vi "lightsheetMain_changeLasers.vi"() -> ()   [LabVIEW 2015]
panel:
  in  "initLaserPower":dbl=2.0
  out "initLasers":T1(array[cluster])=[{"Component ID"="405nm", "COM Port"="COM14", "Type "=enum."omicronLuxX", "init"=1, "Max power (mW)"=60.0}, {"Component ID"="488nm", "COM Port"="COM4", "Type "=enum."omicronLuxX", "init"=1, "Max power (mW)"=60.0}, {"Component ID"="561nm", "COM Port"="COM27", "Type "=enum."coherentObis", "init"=1, "Max power (mW)"=50.0}, {"Component ID"="642nm", "COM Port"="COM12", "Type "=enum."omicronLuxX", "init"=1, "Max power (mW)"=140.0}]
  out "acquisitionTime":u32
  out "opticalSectionThickness (um)":dbl=5.0
  out "acqLaserCOM":refnum<visa-resource-name>[](array[refnum])
  out "acqLaserOff":string[](array[string])
  out "acqLaserOn":string[](array[string])
  out "acqFW":u8[](array[numeric])
  out "Lat x inc (mm)":dbl=0.37273599999999996
  out "Lat y inc (mm)":dbl=0.37273599999999996
  out "no y steps":i32=1
  out "no colours":i32=1
  out "no z imgs (acq)":i32=1
  out "no x steps":i32=1
  out "stop live view":bool
  out "LH yLim (mm)":dbl
  out "RH yLim (mm)":dbl
  in  "Set RH yLim":bool
  in  "Set LH yLim":bool
  out "TH zLim (mm)":dbl
  in  "Set TH zLim":bool
  in  "acqLSFM_3":enum32{"Acquisition (hardware)"}(tab)
  out "Generating tiff stacks":bool
  out "Acquisition in progress":bool
  in  "convertDcimgToTifStacks":bool=TRUE
  in  "setupAcq":bool
  in  "testAcq":bool
  out "x1":dbl
  out "y1":dbl
  out "z1":dbl
  out "x2":dbl
  out "y2":dbl
  out "z2":dbl
  in  "no z steps":i32=1
  in  "% FOV overlap":i32=10
  in  "z inc (um)":dbl=1.0
  in  "642":bool=TRUE
  in  "561":bool=TRUE
  in  "405":bool=TRUE
  in  "488":bool=TRUE
  in  "beginAcq":bool
  in  "stopAcq":bool
  in  "end all comms and exit":bool
  in  "acquisitionMode":enum32{"stop/start  ", "cont."}(radio)
  out "z inc (mm)":dbl=0.01
  in  "Save acq vals":bool
  in  "Read acq vals":bool
  out "Filter wheel":cluster{"FW Handle":u32, "init?":i16}={"FW Handle"=428794912, "init?"=1}
  out "sCMOS":cluster{"init":i16, "sCMOS handle":u32}
  out "Z stage":T2={"System no."=2, "zIdx"=1, "zLim (mm)"=0.0, "0, 1"=0}
  out "XY stage":T3={"System no."=1, "xIdx"=1, "yIdx"=2, "xLim (mm)"=0.0, "yLim (mm)"=0.0, "0, 1"=0}
  in  "LSFM_3":T4(tab)=enum."lasers/filters"
  out "acqDelay (ms)":u32=10
  out "fine axial vel (mm/s)":dbl=10.0
  in  "set axial vel":bool
  in  "filename":string="testImg"
  in  "Index":i32
  in  "Down":bool
  in  "Up":bool
  in  "Left":bool
  in  "Right":bool
  in  "Backward":bool
  in  "Forward":bool
  in  "Axial stepsize (mm/um)":dbl=1.0
  in  "Lateral stepsize (mm/um)":dbl=1.0
  in  "Toggle coarse/fine":enum32{"Coarse (mm) ", "Fine (um) "}(radio)
  out "x (mm)":dbl
  out "y (mm)":dbl
  out "z (mm)":dbl
  in  "Snap img":bool
  in  "set init xy pos":bool
  in  "set fin xy pos":bool
  in  "set init z":bool
  in  "set fin z":bool
  in  "mov init xy":bool
  in  "mov init z":bool
  in  "mov fin xy":bool
  in  "mov fin z":bool
  in  "coarse axial vel (mm/s)":dbl=6.0
  in  "642 nm power (mW)":dbl(slide)=54.0 min=0.0 max=60.0 step=1.0 scale=0.0..140.0
  in  "561 nm power (mW)":dbl(slide)=8.0 min=0.0 max=60.0 step=1.0 scale=0.0..60.0
  in  "488 nm power (mW)":dbl(slide)=5.0 min=0.0 max=60.0 step=1.0 scale=0.0..60.0
  in  "405 nm power (mW)":dbl(slide)=5.0 min=0.0 max=60.0 step=1.0 scale=0.0..60.0
  in  "FW pos":u16(ring)=4 items=["460/36 [DAPI]"=1, "525/50 [FITC]"=2, "605/70 [Cy3]"=3, "665/LP [Cy5]"=4, "Empty-1"=5, "Empty-2"=6]
  in  "next":bool
  in  "prev":bool
  in  "642 nm ON":bool
  in  "642 nm OFF":bool
  in  "561 nm ON":bool
  in  "561 nm OFF":bool
  in  "488 nm ON":bool
  in  "488 nm OFF":bool
  in  "405 nm ON":bool
  in  "405 nm OFF":bool
  in  "405 filter":u8(ring)=1 items=["460/36 [DAPI]"=1, "525/50 [FITC]"=2, "605/70 [Cy3]"=3, "665/LP [Cy5]"=4, "Empty-1"=5, "Empty-2"=6]
  in  "488 filter":u8(ring)=2 items=["460/36 [DAPI]"=1, "525/50 [FITC]"=2, "605/70 [Cy3]"=3, "665/LP [Cy5]"=4, "Empty-1"=5, "Empty-2"=6]
  in  "561 filter":u8(ring)=3 items=["460/36 [DAPI]"=1, "525/50 [FITC]"=2, "605/70 [Cy3]"=3, "665/LP [Cy5]"=4, "Empty-1"=5, "Empty-2"=6]
  in  "642 filter":u8(ring)=4 items=["460/36 [DAPI]"=1, "525/50 [FITC]"=2, "605/70 [Cy3]"=3, "665/LP [Cy5]"=4, "Empty-1"=5, "Empty-2"=6]
  out "Acquiring?":bool
  in  "live stream":bool
  in  "Set exp. time":bool
  in  "Exposure time (s)":dbl=1.0
  in  "stop live stream":bool
  in  "View stream":bool=TRUE
  out "Img. pixel size":dbl=0.26
  out "No. of pix":u16=2048
  in  "pixel binning":u16(ring) items=["1x1"=1, "2x2"=2, "4x4"=4]
  in  "No. pix":u16=2048
  in  "scmos pixel size (um)":dbl=6.5 format="%#_13g"
  out "FOV (mm)":dbl=0.53248
  in  "sensorSize":dbl=13.312 format="%#_13g"
  in  "Mag":dbl=25.0 format="%#_13g"
  in  "z":bool
  in  "xy":bool
  in  "488nm":bool=TRUE
  in  "405nm":bool=TRUE
  in  "561nm":bool=TRUE
  in  "642nm":bool=TRUE
  in  "sCMOS":bool
  in  "FW":bool=TRUE
  out "Appended path":path=path "C:/Users/LSFM_2/Desktop/dataAcq_2705/bothIllAxis/4umBead0.tif"
  in  "Base path":path=path "C:/Users/sims01/Desktop/dataAcq"
  in  "dcimgToStack":bool
  in  "stageAccDelay (ms)":u32
  # "Stage limits"
  # "Positions"
  # "Step sizes"
  # "Currrent positions"
  # "Motion control"
  # "Move stages"
  # "lasers"
  # "filters"
  # "File setup"
  # "Hardware initialization"
  # "Microscope properties"
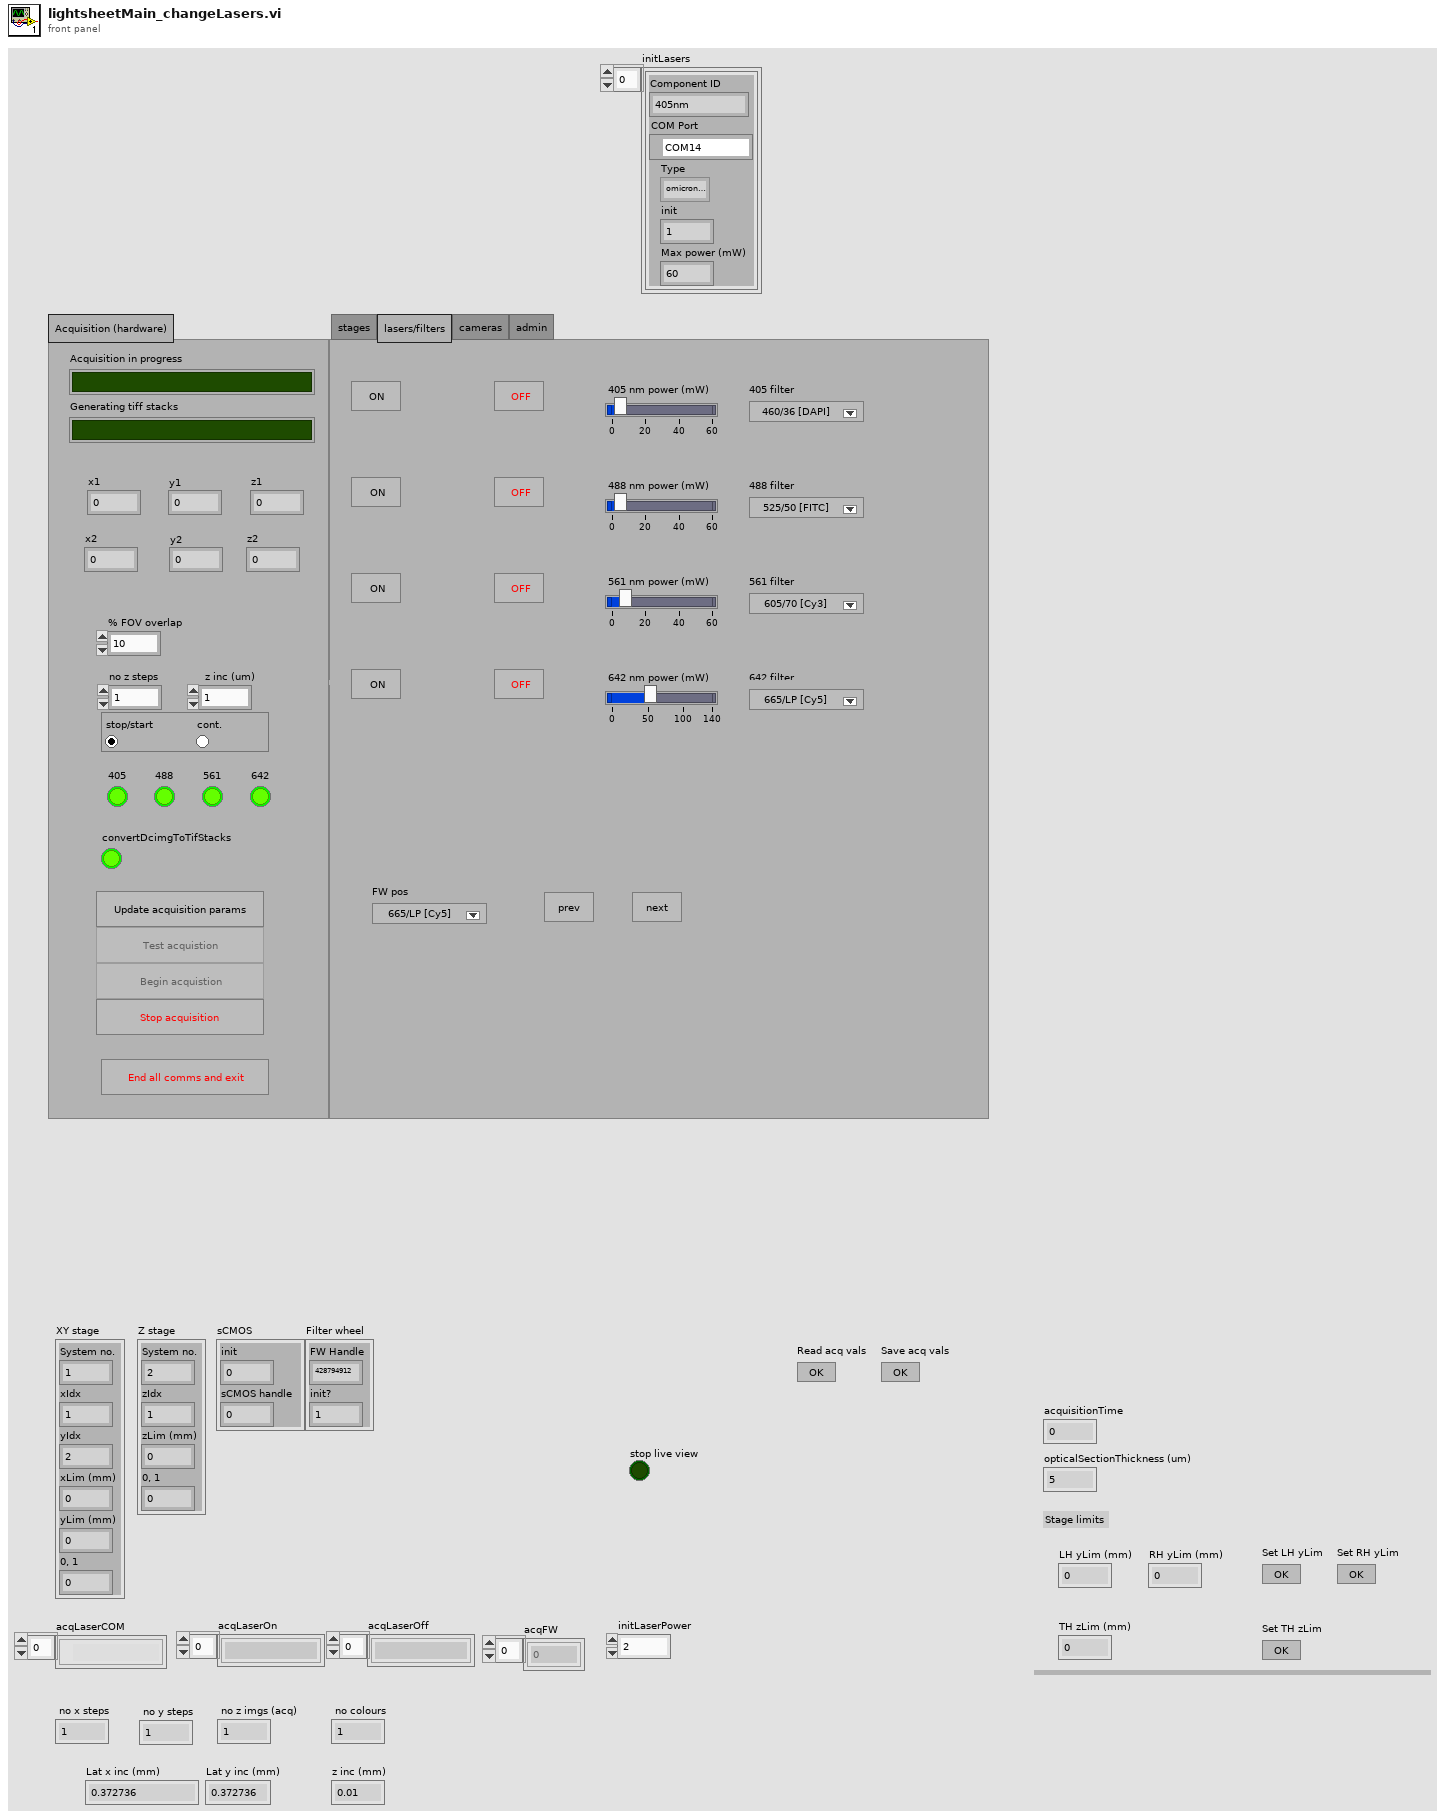
[diagram p1: front panel]
types:
  T1 = cluster{"Component ID":string, "COM Port":refnum<visa-resource-name>, "Type ":enum16{"omicronLuxX", "coherentObis"}, "init":i16, "Max power (mW)":dbl}[]
  T2 = cluster{"System no.":i32, "zIdx":i32, "zLim (mm)":dbl, "0, 1":i16}
  T3 = cluster{"System no.":i32, "xIdx":i32, "yIdx":i32, "xLim (mm)":dbl, "yLim (mm)":dbl, "0, 1":i16}
  T4 = enum32{"stages", "lasers/filters", "cameras", "admin"}
  T5 = enum8{"Enabled", "Disabled", "Disabled and Grayed Out"}
  T6 = cluster{"Component ID":string, "COM Port":refnum<visa-resource-name>, "Type ":enum16{"omicronLuxX", "coherentObis"}, "init":i16, "Max power (mW)":dbl}
  T7 = enum32{"Invalid", "Standard", "Closed", "Hidden", "Minimized", "Maximized"}
  T8 = cluster{"height":u32, "width":u32, "datatype":u32}
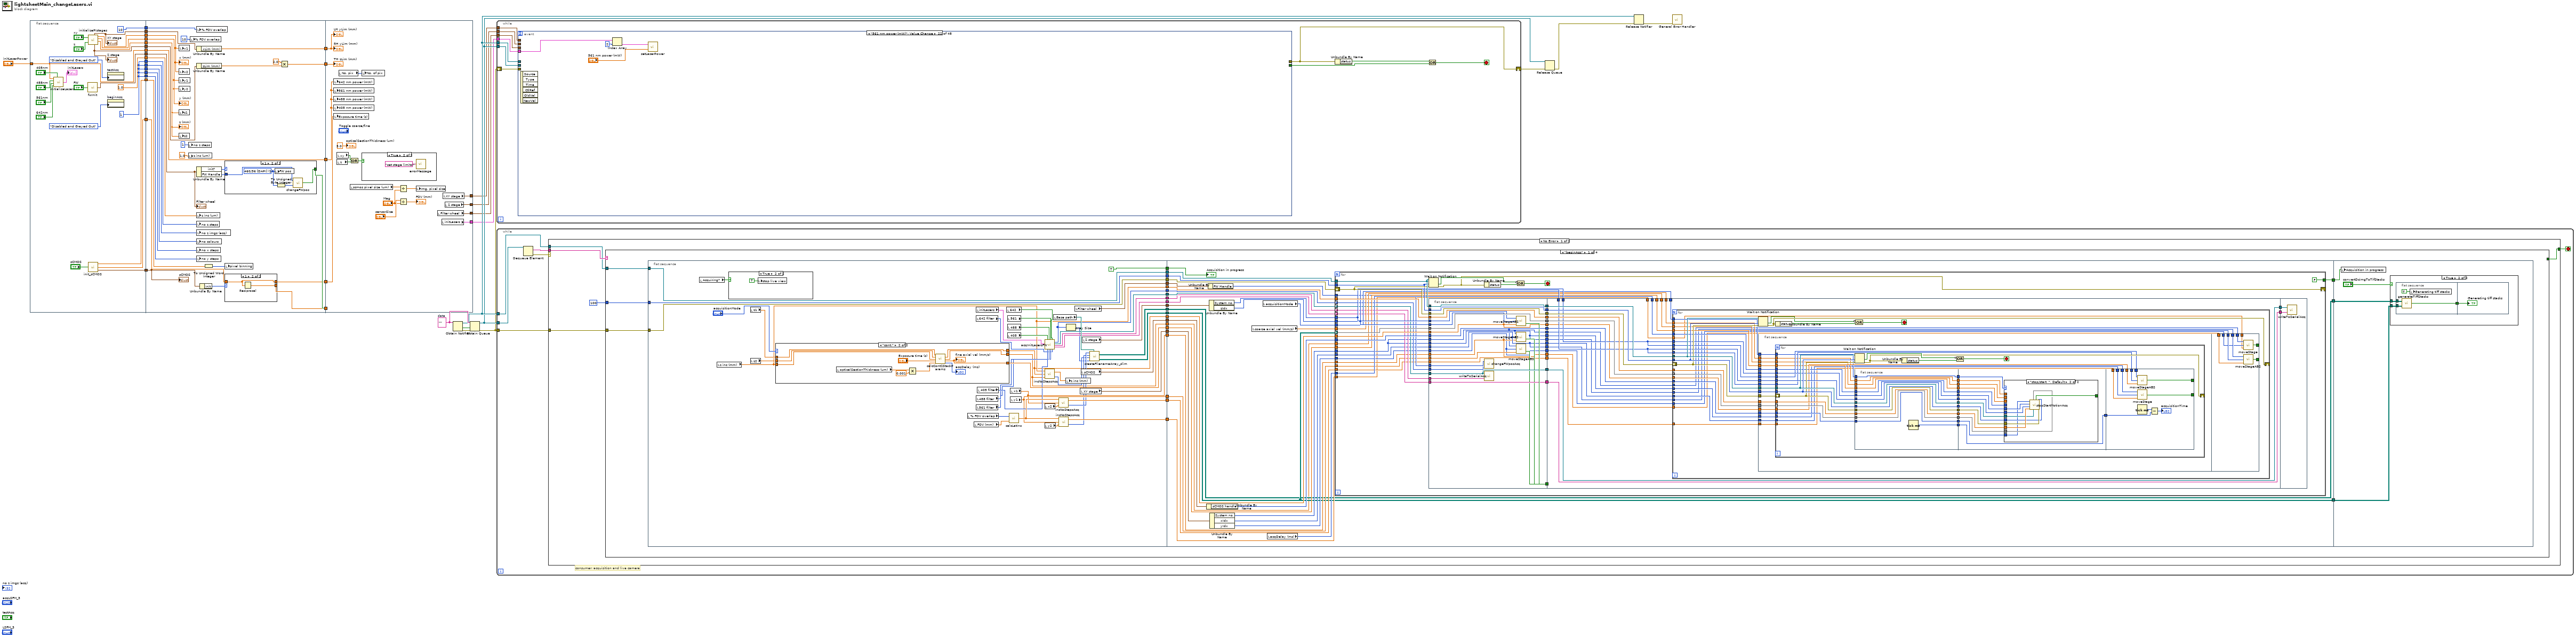
[diagram p0: block diagram]
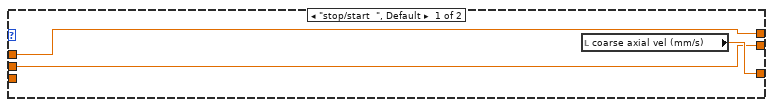
[diagram p3: hidden frame]
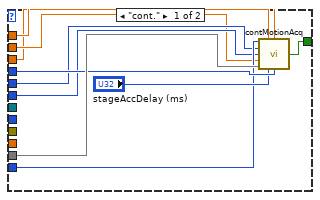
[diagram p4: hidden frame]
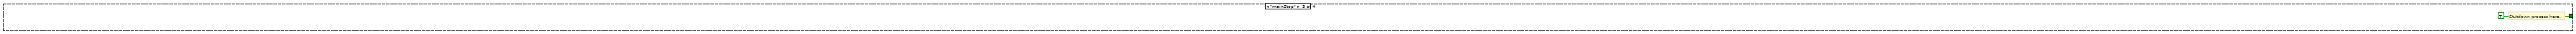
[diagram p7: hidden frame]
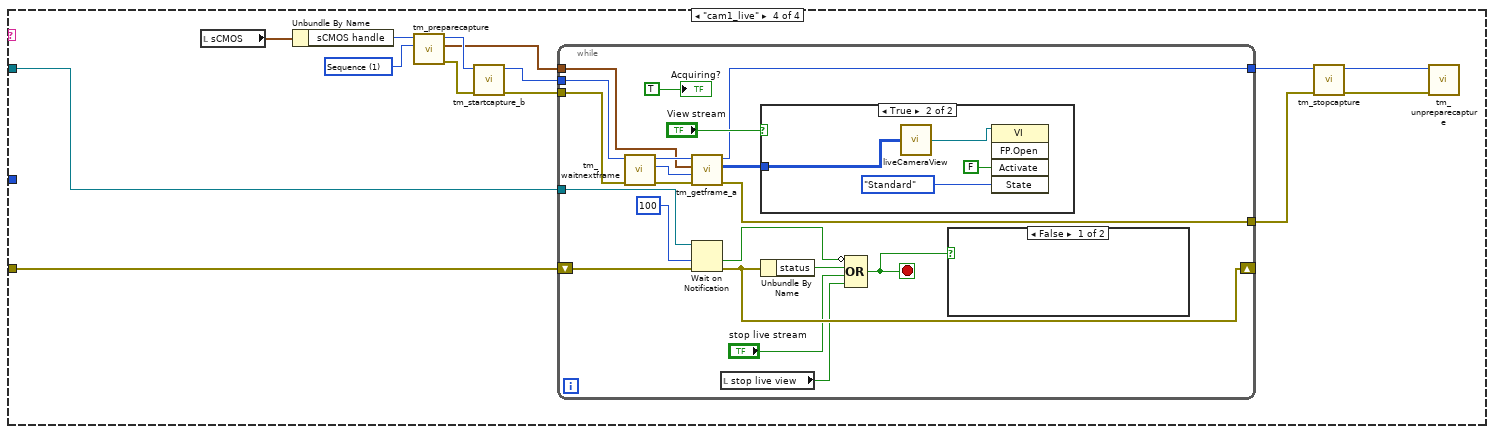
[diagram p8: hidden frame]
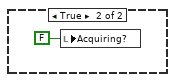
[diagram p9: hidden frame]
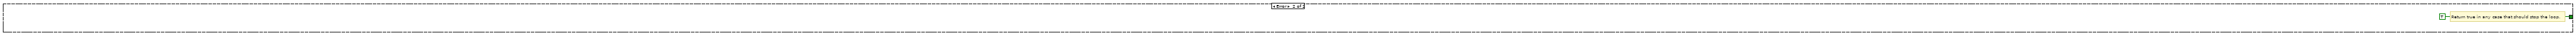
[diagram p11: hidden frame]
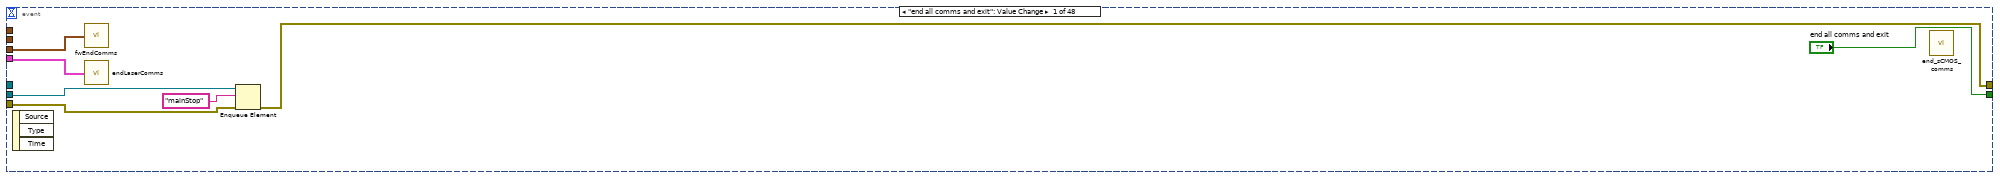
[diagram p12: hidden frame]
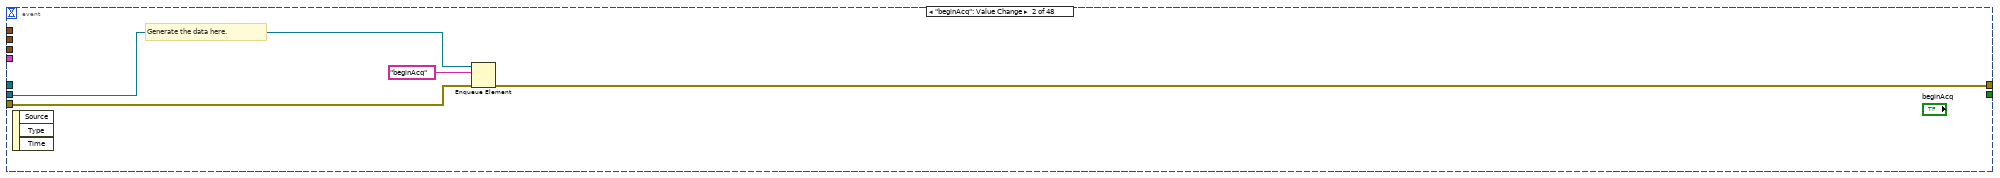
[diagram p13: hidden frame]
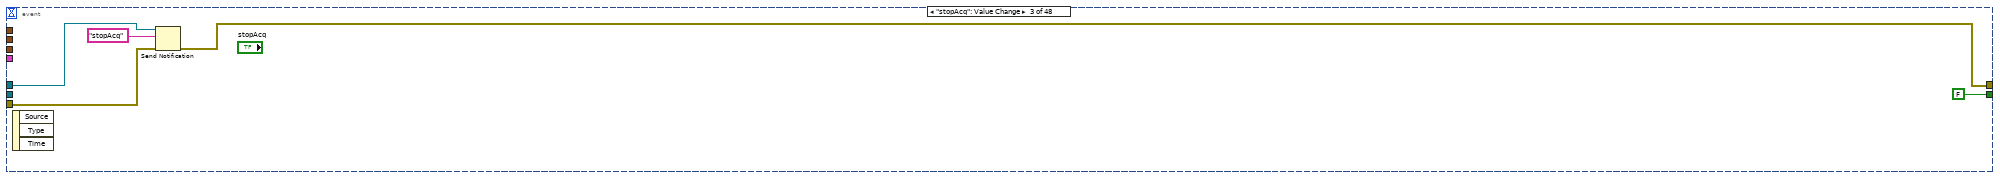
[diagram p14: hidden frame]
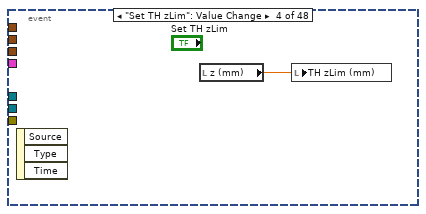
[diagram p15: hidden frame]
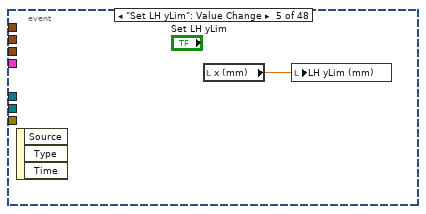
[diagram p16: hidden frame]
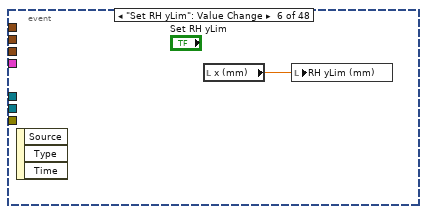
[diagram p17: hidden frame]
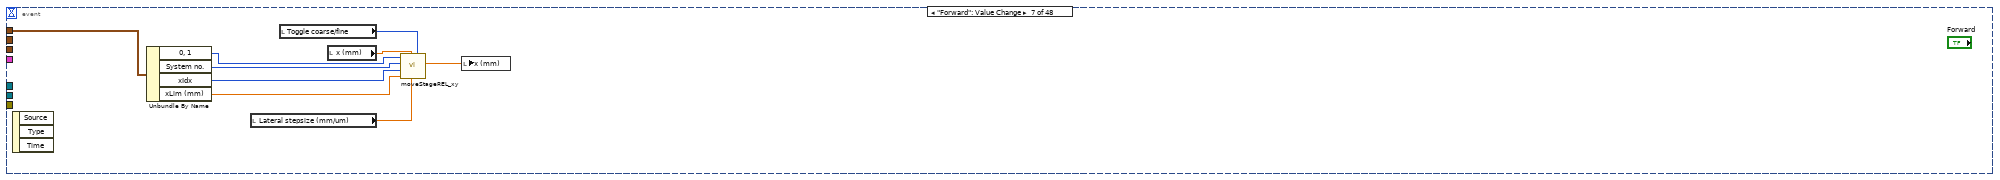
[diagram p18: hidden frame]
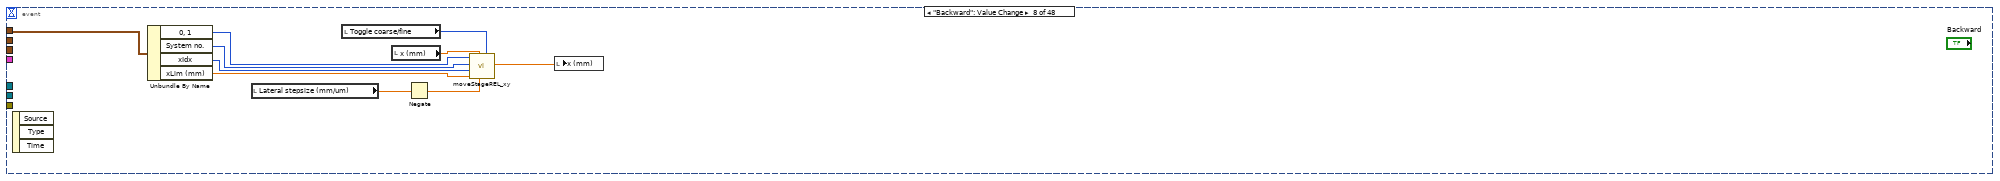
[diagram p19: hidden frame]
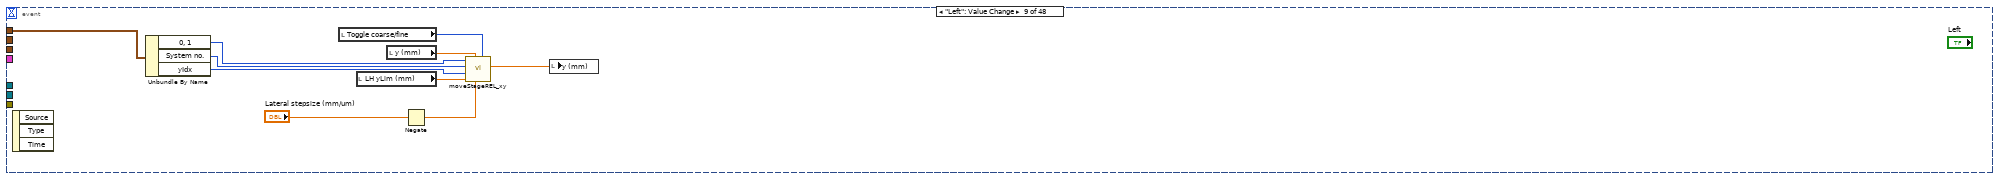
[diagram p20: hidden frame]
diagram:
  w26 = ""  # data
  n1 = flat-sequence {
    tunnel: [w59] -> w37
    tunnel: [w58] -> w36
    tunnel: [w57] -> w35
    tunnel: [w50] -> w34
    tunnel: [w49] -> w33
    tunnel: [w56] -> w32
    tunnel: [w55] -> w16
    tunnel: [w54] -> w15
    tunnel: [w48] -> w11
    tunnel: [w46] -> w10
    tunnel: [w46] -> w9
    tunnel: [w46] -> w8
    tunnel: [w46] -> w7
    tunnel: [10 ("% FOV overlap")] -> w6
    tunnel: [w46] -> w5
    tunnel: [1.0 ("z inc (um)")] -> w4
    tunnel: "initLaserPower" -> [w38]
    tunnel: [w38] -> w1
    tunnel: w37 -> [w75]
    tunnel: w36 -> [w76]
    tunnel: w35 -> [w77]
    tunnel: w34 -> [w90]
    tunnel: w33 -> [w92]
    tunnel: w32 -> [w89]
    tunnel: [w86] -> w31
    tunnel: [w85] -> w30
    tunnel: [w84] -> w29
    tunnel: w16 -> [w83]
    tunnel: w15 -> [w82]
    tunnel: [w81] -> w14
    tunnel: [w80] -> w13
    tunnel: w11 -> [w71]
    tunnel: w10 -> [w70]
    tunnel: w9 -> [w69]
    tunnel: w8 -> [w68]
    tunnel: w7 -> [w67]
    tunnel: w6 -> [w66]
    tunnel: w5 -> [w65]
    tunnel: w4 -> [w64]
    tunnel: [w62] -> w3
    tunnel: w1 -> [w62]
    tunnel: w31 -> [_]
    tunnel: w30 -> [w113]
    tunnel: w29 -> [_]
    tunnel: [w112] -> w18
    tunnel: [w111] -> w17
    tunnel: [w110] -> w19
    tunnel: w14 -> [w109]
    tunnel: w13 -> [w108]
    tunnel: [w102] -> w12
    tunnel: w3 -> [w101]
    frame #0 {
      w46 = 1 ("no y steps")
      n2 = call "initialiseLasers.vi"("initLaserPower"=w38, "488 nm"="488nm", "561 nm"="561nm", "642 nm"="642nm", "405 nm"="405nm") -> ("outputLasers"=→"initLasers":T1)
      n3 = call "fwInit.vi"("FW init?"="FW") -> ("Filter wheel init"=w56:cluster{"FW Handle":u32, "init?":i16})
      n4 = call "initializePIstages.vi"("xy stage"="xy", "z stage"="z") -> ("XY stage"=w54:T3, "Z stage"=w55:T2, "current xPos (mm)"=w59:dbl, "current yPos (mm)"=w58:dbl, "current zPos (mm)"=w57:dbl)  [unwired: 1 in]
      "XY stage" <- w54
      "Z stage" <- w55
      n5 = call "init_sCMOS.vi"("sCMOS_1"="sCMOS") -> ("Binning"=w48:dbl, "Exposure"=w50:dbl, "sCMOS init"=w49:cluster{"init":i16, "sCMOS handle":u32})
      n6 = property on="testAcq" class="Bool"("DisabledEnum"=T5."Disabled and Grayed Out" ("Disabled")) -> ()  [unwired: 2 in, 2 out]
      n7 = property on="beginAcq" class="Bool"("DisabledEnum"=T5."Disabled and Grayed Out" ("Disabled")) -> ()  [unwired: 2 in, 2 out]
    }
    frame #1 {
      n8 = local write "x1"(w75) -> ()
      n9 = local write "x2"(w75) -> ()
      n10 = local write "y1"(w76) -> ()
      n11 = local write "y2"(w76) -> ()
      n12 = local write "z1"(w77) -> ()
      n13 = local write "z2"(w77) -> ()
      n14 = local write "no z steps"(1 ("no z steps")) -> ()
      n15 = local write "z inc (um)"(1.0 ("z inc (um)")) -> ()
      n16 = local write "% FOV overlap"(10 ("% FOV overlap")) -> ()
      n17 = local write "% FOV overlap"(w66) -> ()
      n18 = Unbundle By Name(w82) -> ("xLim (mm)"=w81:dbl)
      n19 = Unbundle By Name(w83) -> ("zLim (mm)"=w79:dbl)
      n20 = Unbundle By Name(w89) -> ("init?"=w88:i16, "FW Handle"=w87:u32)
      n21 = local write "z inc (um)"(w64) -> ()
      n22 = local write "no z steps"(w65) -> ()
      n23 = local write "no z imgs (acq)"(w68) -> ()
      n24 = local write "no colours"(w69) -> ()
      n25 = local write "no x steps"(w67) -> ()
      n26 = local write "no y steps"(w70) -> ()
      n27 = Unbundle By Name(w92) -> ("init"=w91:i16)
      n28 = To Unsigned Word Integer(number=w71) -> (unsigned 16bit integer=w72:u16)
      n29 = case shown="1" w88 {
        tunnel: w87 -> [_ w97]
        tunnel: [FALSE ("fwPosChanged") w96] -> w86
        frame 0, Default {
        }
        frame 1 {
          w94 = u16 1 items=["460/36 [DAPI]"=1, "525/50 [FITC]"=2, "605/70 [Cy3]"=3, "665/LP [Cy5]"=4, "Empty-1"=5, "Empty-2"=6] ("Filter wheel position")
          n30 = local write "FW pos"(w94) -> ()
          n31 = To Unsigned Byte Integer(number=w94) -> (unsigned 8bit integer=w95:u8)
          n32 = call "changeFWpos.vi"("FW pos"=w95, "FWhandle"=w97) -> ("fwPosChanged"=w96:bool)
        }
      }
      n33 = local write "pixel binning"(w72) -> ()
      n34 = case shown="1" w91 {
        tunnel: w90 -> [_ w100]
        tunnel: [w98 w100] -> w85
        tunnel: [w98 w99] -> w84
        frame 0, Default {
          w98 = 1.0
        }
        frame 1 {
          n35 = Reciprocal(x=w100) -> (1/x=w99:dbl)
        }
      }
      n36 = Multiply(x=2.0, y=w79) -> (x*y=w80:dbl)
      "z (mm)" <- w77
      "y (mm)" <- w76
      "x (mm)" <- w75
      "sCMOS" <- w92
      "Filter wheel" <- w89
    }
    frame #2 {
      n37 = local write "642 nm power (mW)"(w101) -> ()
      n38 = local write "561 nm power (mW)"(w101) -> ()
      n39 = local write "488 nm power (mW)"(w101) -> ()
      n40 = local write "405 nm power (mW)"(w101) -> ()
      n41 = local write "Exposure time (s)"(w113) -> ()
      n42 = local read "xy"() -> (w115:bool)
      n43 = local read "z"() -> (w114:bool)
      n44 = local read "No. pix"() -> (w104:u16)
      n45 = Or(x=w115, y=w114) -> (x .or. y?=w116:bool)
      n46 = local read "scmos pixel size (um)"() -> (w106:dbl)
      n47 = local write "No. of pix"(w104) -> ()
      n48 = case shown="True" w116 {
        frame False {
        }
        frame True {
          n49 = call "errorMessage.vi"("messageText"="set stage limits!") -> ()  [unwired: 3 out]
        }
      }
      n50 = Divide(x=w106, y="Mag") -> (x/y=w105:dbl)
      n51 = Divide(x="sensorSize", y="Mag") -> (x/y=→"FOV (mm)":dbl)
      n52 = local write "Img. pixel size"(w105) -> ()
      n53 = local read "Filter wheel"() -> (w112:cluster{"FW Handle":u32, "init?":i16})
      n54 = local read "initLasers"() -> (w102:T1)
      n55 = local read "XY stage"() -> (w111:T3)
      n56 = local read "Z stage"() -> (w110:T2)
      "TH zLim (mm)" <- w108
      "RH yLim (mm)" <- w109
      "LH yLim (mm)" <- w109
      "opticalSectionThickness (um)" <- 5.0 ("opticalSectionThickness (um)")
    }
  }
  n57 = Obtain Notifier(notification data type=w26) -> (notifier out=w22:refnum<notifier>, created new?=w28:bool, error out=w27:errorcluster)  [unwired: 3 in]
  n58 = Obtain Queue(element data type=w26, create if not found? (T)=w28, error in (no error)=w27) -> (queue out=w21:refnum<queue>, error out=w20:errorcluster)  [unwired: 2 in, 1 out]
  n59 = while {
    shift-right: [w126] -> w25
    shift-left: w20 -> [w129]
    tunnel: w21 -> [w130]
    tunnel: w22 -> [w124]
    tunnel: w19 -> [w123]
    tunnel: w18 -> [w122]
    tunnel: w17 -> [w121]
    tunnel: w12 -> [w120]
    stop <- w127 stop-if-true
    n60 = event shown="[21] \"561 nm power (mW)\": Value Change" {
      selector: _ -> [_ _ _ _ _ _ _ _ _ _ _ _ _ _ _ _ _ _ _ _ _ _ _ _ _ _ _ _ _ _ _ _ _ _ _ _ _ _ _ _ _ _ _ _ _ _ _ _]
      dyn-events: _ -> [_ _ _ _ _ _ _ _ _ _ _ _ _ _ _ _ _ _ _ _ _ _ _ _ _ _ _ _ _ _ _ _ _ _ _ _ _ _ _ _ _ _ _ _ _ _ _ _]
      timeout: _ -> [_ _ _ _ _ _ _ _ _ _ _ _ _ _ _ _ _ _ _ _ _ _ _ _ _ _ _ _ _ _ _ _ _ _ _ _ _ _ _ _ _ _ _ _ _ _ _ _]
      tunnel: w130 -> [w134 w141 _ _ _ _ _ _ _ _ _ _ _ _ _ _ _ _ _ _ _ _ _ _ _ _ _ _ _ w306 _ _ _ _ _ _ _ _ _ _ _ _ _ _ _ _ _ _]
      tunnel: w129 -> [w136 w140 w146 _ _ _ _ _ _ _ _ _ _ _ _ _ _ _ _ _ _ _ _ _ _ _ _ _ _ w308 _ _ _ _ _ _ _ _ _ _ _ _ _ _ _ _ _ _]
      tunnel: [w135 w139 w145 _ _ _ _ _ _ _ _ _ _ _ _ _ _ _ _ _ _ _ _ _ _ _ _ _ _ w307 _ _ _ _ _ _ _ _ _ _ _ _ _ _ _ _ _ _] -> w126
      tunnel: ["end all comms and exit" _ FALSE ("stop") _ _ _ _ _ _ _ _ _ _ _ _ _ _ _ _ _ _ _ _ _ _ _ _ _ _ _ _ _ _ _ _ _ _ _ _ _ _ _ _ _ _ _ _ _] -> w128
      tunnel: w124 -> [_ _ w144 _ _ _ _ _ _ _ _ _ _ _ _ _ _ _ _ _ _ _ _ _ _ _ _ _ _ _ _ _ _ _ _ _ _ _ _ _ _ _ _ _ _ _ _ _]
      tunnel: w123 -> [_ _ _ _ _ _ _ _ _ _ w196 w206 w208 _ _ _ _ _ _ _ _ _ _ _ _ _ _ _ _ _ _ _ _ _ _ _ _ _ _ w376 w380 _ _ _ _ _ w417 _]
      tunnel: w122 -> [w131 _ _ _ _ _ _ _ _ _ _ _ _ w211 _ _ w224 _ _ w240 _ _ w255 _ _ w271 w277 w288 _ _ _ _ _ _ _ _ _ _ _ _ _ _ _ _ _ _ w418 _]
      tunnel: w121 -> [_ _ _ _ _ _ w158 w168 w178 w187 _ _ _ _ _ _ _ _ _ _ _ _ _ _ _ _ _ _ _ _ _ _ _ _ _ w355 w356 _ _ _ _ _ _ _ _ _ w416 _]
      tunnel: w120 -> [w132 _ _ _ _ _ _ _ _ _ _ _ _ w213 w217 w222 w228 w232 w237 w243 w247 w252 w258 w262 w267 _ _ _ _ _ _ _ _ _ _ _ _ _ _ _ _ _ _ _ _ _ w414 _]
      event "end all comms and exit": Value Change {
        n61 = event-data() -> ()  [unwired: 1 in, 3 out]
        n62 = call "fwEndComms.vi"("fw cluster"=w131) -> ()
        n63 = call "endLaserComms.vi"("outputLasers"=w132) -> ()
        n64 = Enqueue Element(queue=w134, element="mainStop", error in (no error)=w136) -> (error out=w135:errorcluster)  [unwired: 1 in, 2 out]
        n65 = call "end_sCMOS_comms.vi"() -> ()  [unwired: 1 in]
      }
      event "beginAcq": Value Change {
        # "Generate the data here."
        n66 = event-data() -> ()  [unwired: 1 in, 3 out]
        n67 = Enqueue Element(queue=w141, element="beginAcq", error in (no error)=w140) -> (error out=w139:errorcluster)  [unwired: 1 in, 2 out]
      }
      event "stopAcq": Value Change {
        n68 = event-data() -> ()  [unwired: 1 in, 3 out]
        n69 = Send Notification(notification="stopAcq", notifier=w144, error in (no error)=w146) -> (error out=w145:errorcluster)  [unwired: 1 out]
      }
      event "Set TH zLim": Value Change {
        n70 = event-data() -> ()  [unwired: 1 in, 3 out]
        n71 = local read "z (mm)"() -> (w147:dbl)
        n72 = local write "TH zLim (mm)"(w147) -> ()
      }
      event "Set LH yLim": Value Change {
        n73 = event-data() -> ()  [unwired: 1 in, 3 out]
        n74 = local read "x (mm)"() -> (w148:dbl)
        n75 = local write "LH yLim (mm)"(w148) -> ()
      }
      event "Set RH yLim": Value Change {
        n76 = event-data() -> ()  [unwired: 1 in, 3 out]
        n77 = local read "x (mm)"() -> (w149:dbl)
        n78 = local write "RH yLim (mm)"(w149) -> ()
      }
      event "Forward": Value Change {
        n79 = event-data() -> ()  [unwired: 1 in, 3 out]
        n80 = Unbundle By Name(w158) -> ("0, 1"=w157:i16, "System no."=w156:i32, "xIdx"=w155:i32, "xLim (mm)"=w154:dbl)
        n81 = local read "Lateral stepsize (mm/um)"() -> (w153:dbl)
        n82 = local read "Toggle coarse/fine"() -> (w151:enum32{"Coarse (mm) ", "Fine (um) "})
        n83 = local read "x (mm)"() -> (w152:dbl)
        n84 = call "moveStageREL_xy.vi"("Radio Buttons"=w151, "increment"=w153, "initPos (mm)"=w152, "stage lim (mm)"=w154, "axisIdx"=w155, "System no."=w156, "stageInit"=w157) -> ("finPos"=w150:dbl)  [unwired: 3 in]
        n85 = local write "x (mm)"(w150) -> ()
      }
      event "Backward": Value Change {
        n86 = event-data() -> ()  [unwired: 1 in, 3 out]
        n87 = Unbundle By Name(w168) -> ("0, 1"=w167:i16, "System no."=w166:i32, "xIdx"=w165:i32, "xLim (mm)"=w164:dbl)
        n88 = local read "Lateral stepsize (mm/um)"() -> (w163:dbl)
        n89 = local read "Toggle coarse/fine"() -> (w161:enum32{"Coarse (mm) ", "Fine (um) "})
        n90 = local read "x (mm)"() -> (w160:dbl)
        n91 = Negate(x=w163) -> (-x=w162:dbl)
        n92 = call "moveStageREL_xy.vi"("Radio Buttons"=w161, "increment"=w162, "initPos (mm)"=w160, "stage lim (mm)"=w164, "axisIdx"=w165, "System no."=w166, "stageInit"=w167) -> ("finPos"=w159:dbl)  [unwired: 3 in]
        n93 = local write "x (mm)"(w159) -> ()
      }
      event "Left": Value Change {
        n94 = event-data() -> ()  [unwired: 1 in, 3 out]
        n95 = Unbundle By Name(w178) -> ("0, 1"=w176:i16, "System no."=w175:i32, "yIdx"=w174:i32)
        n96 = local read "Toggle coarse/fine"() -> (w171:enum32{"Coarse (mm) ", "Fine (um) "})
        n97 = local read "LH yLim (mm)"() -> (w173:dbl)
        n98 = local read "y (mm)"() -> (w170:dbl)
        n99 = Negate(x="Lateral stepsize (mm/um)") -> (-x=w172:dbl)
        n100 = call "moveStageREL_xy.vi"("Radio Buttons"=w171, "increment"=w172, "initPos (mm)"=w170, "stage lim (mm)"=w173, "axisIdx"=w174, "System no."=w175, "stageInit"=w176) -> ("finPos"=w169:dbl)  [unwired: 3 in]
        n101 = local write "y (mm)"(w169) -> ()
      }
      event "Right": Value Change {
        n102 = event-data() -> ()  [unwired: 1 in, 3 out]
        n103 = Unbundle By Name(w187) -> ("0, 1"=w185:i16, "System no."=w184:i32, "yIdx"=w183:i32)
        n104 = local read "Lateral stepsize (mm/um)"() -> (w180:dbl)
        n105 = local read "Toggle coarse/fine"() -> (w179:enum32{"Coarse (mm) ", "Fine (um) "})
        n106 = local read "RH yLim (mm)"() -> (w182:dbl)
        n107 = local read "y (mm)"() -> (w181:dbl)
        n108 = call "moveStageREL_xy.vi"("Radio Buttons"=w179, "increment"=w180, "initPos (mm)"=w181, "stage lim (mm)"=w182, "axisIdx"=w183, "System no."=w184, "stageInit"=w185) -> ("finPos"=w186:dbl)  [unwired: 3 in]
        n109 = local write "y (mm)"(w186) -> ()
      }
      event "Up": Value Change {
        n110 = event-data() -> ()  [unwired: 1 in, 4 out]
        n111 = Unbundle By Name(w196) -> ("0, 1"=w195:i16, "System no."=w194:i32, "zIdx"=w193:i32)
        n112 = local read "Toggle coarse/fine"() -> (w189:enum32{"Coarse (mm) ", "Fine (um) "})
        n113 = local read "TH zLim (mm)"() -> (w192:dbl)
        n114 = local read "z (mm)"() -> (w191:dbl)
        n115 = call "moveStageREL_z.vi"("Radio Buttons"=w189, "increment"="Axial stepsize (mm/um)", "initPos (mm)"=w191, "stage lim (mm)"=w192, "axisIdx"=w193, "System no."=w194, "stageInit"=w195) -> ("finPos"=w190:dbl)  [unwired: 3 in]
        n116 = local write "z (mm)"(w190) -> ()
      }
      event "Down": Value Change {
        n117 = event-data() -> ()  [unwired: 1 in, 4 out]
        n118 = Unbundle By Name(w206) -> ("0, 1"=w204:i16, "System no."=w203:i32, "zIdx"=w202:i32)
        n119 = local read "Axial stepsize (mm/um)"() -> (w205:dbl)
        n120 = local read "Toggle coarse/fine"() -> (w200:enum32{"Coarse (mm) ", "Fine (um) "})
        n121 = local read "TH zLim (mm)"() -> (w197:dbl)
        n122 = local read "z (mm)"() -> (w199:dbl)
        n123 = Negate(x=w205) -> (-x=w201:dbl)
        n124 = call "moveStageREL_z.vi"("Radio Buttons"=w200, "increment"=w201, "initPos (mm)"=w199, "stage lim (mm)"=w197, "axisIdx"=w202, "System no."=w203, "stageInit"=w204) -> ("finPos"=w198:dbl)  [unwired: 3 in]
        n125 = local write "z (mm)"(w198) -> ()
      }
      event "set axial vel": Value Change {
        n126 = event-data() -> ()  [unwired: 1 in, 6 out]
        n127 = call "setVel.vi"("vel (mm/s)"="coarse axial vel (mm/s)", "input cluster"=w208) -> ()
      }
      event "405 nm ON": Value Change {
        n128 = event-data() -> ()  [unwired: 1 in, 6 out]
        n129 = Index Array(array=w213, index=0) -> (element=w212:T6)
        n130 = call "changeLaserFW.vi"("FW pos"="405 filter", "inputFW"=w211, "inputLaser"=w212) -> ("changePos?"=w210:i16)
        n131 = case shown="0, Default" w210 {
          tunnel: "405 filter" -> [_ w216]
          frame 0, Default {
          }
          frame 1 {
            n132 = To Unsigned Word Integer(number=w216) -> (unsigned 16bit integer=w215:u16)
            n133 = local write "FW pos"(w215) -> ()
          }
        }
      }
      event "405 nm OFF": Value Change {
        n134 = event-data() -> ()  [unwired: 1 in, 6 out]
        n135 = Index Array(array=w217, index=0) -> (element=w219:T6)
        n136 = call "turnLaserOff.vi"("input cluster"=w219) -> ()  [unwired: 1 out]
      }
      event "405 nm power (mW)": Value Change {
        n137 = event-data() -> ()  [unwired: 1 in, 6 out]
        n138 = Index Array(array=w222, index=0) -> (element=w221:T6)
        n139 = call "setLaserPower.vi"("laser power (mW)"="405 nm power (mW)", "laser"=w221) -> ()  [unwired: 1 out]
        n140 = call "setLaserPower.vi"() -> ()  [unwired: 2 in, 1 out]
      }
      event "488 nm ON": Value Change {
        n141 = event-data() -> ()  [unwired: 1 in, 6 out]
        n142 = Index Array(array=w228, index=1) -> (element=w226:T6)
        n143 = call "changeLaserFW.vi"("FW pos"="488 filter", "inputFW"=w224, "inputLaser"=w226) -> ("changePos?"=w227:i16)
        n144 = case shown="0, Default" w227 {
          tunnel: "488 filter" -> [_ w231]
          frame 0, Default {
          }
          frame 1 {
            n145 = To Unsigned Word Integer(number=w231) -> (unsigned 16bit integer=w230:u16)
            n146 = local write "FW pos"(w230) -> ()
          }
        }
      }
      event "488 nm OFF": Value Change {
        n147 = event-data() -> ()  [unwired: 1 in, 6 out]
        n148 = Index Array(array=w232, index=1) -> (element=w233:T6)
        n149 = call "turnLaserOff.vi"("input cluster"=w233) -> ()  [unwired: 1 out]
      }
      event "488 nm power (mW)": Value Change {
        n150 = event-data() -> ()  [unwired: 1 in, 6 out]
        n151 = Index Array(array=w237, index=1) -> (element=w236:T6)
        n152 = call "setLaserPower.vi"("laser power (mW)"="488 nm power (mW)", "laser"=w236) -> ()  [unwired: 1 out]
      }
      event "561 nm ON": Value Change {
        n153 = event-data() -> ()  [unwired: 1 in, 6 out]
        n154 = Index Array(array=w243, index=2) -> (element=w241:T6)
        n155 = call "changeLaserFW.vi"("FW pos"="561 filter", "inputFW"=w240, "inputLaser"=w241) -> ("changePos?"=w242:i16)
        n156 = case shown="0, Default" w242 {
          tunnel: "561 filter" -> [_ w246]
          frame 0, Default {
          }
          frame 1 {
            n157 = To Unsigned Word Integer(number=w246) -> (unsigned 16bit integer=w245:u16)
            n158 = local write "FW pos"(w245) -> ()
          }
        }
      }
      event "561 nm OFF": Value Change {
        n159 = event-data() -> ()  [unwired: 1 in, 6 out]
        n160 = Index Array(array=w247, index=2) -> (element=w248:T6)
        n161 = call "turnLaserOff.vi"("input cluster"=w248) -> ()  [unwired: 1 out]
      }
      event "561 nm power (mW)": Value Change {
        n162 = event-data() -> ()  [unwired: 1 in, 6 out]
        n163 = Index Array(array=w252, index=2) -> (element=w251:T6)
        n164 = call "setLaserPower.vi"("laser power (mW)"="561 nm power (mW)", "laser"=w251) -> ()  [unwired: 1 out]
      }
      event "642 nm ON": Value Change {
        n165 = event-data() -> ()  [unwired: 1 in, 6 out]
        n166 = Index Array(array=w258, index=3) -> (element=w256:T6)
        n167 = call "changeLaserFW.vi"("FW pos"="642 filter", "inputFW"=w255, "inputLaser"=w256) -> ("changePos?"=w257:i16)
        n168 = case shown="0, Default" w257 {
          tunnel: "642 filter" -> [_ w261]
          frame 0, Default {
          }
          frame 1 {
            n169 = To Unsigned Word Integer(number=w261) -> (unsigned 16bit integer=w260:u16)
            n170 = local write "FW pos"(w260) -> ()
          }
        }
      }
      event "642 nm OFF": Value Change {
        n171 = event-data() -> ()  [unwired: 1 in, 6 out]
        n172 = Index Array(array=w262, index=3) -> (element=w263:T6)
        n173 = call "turnLaserOff.vi"("input cluster"=w263) -> ()  [unwired: 1 out]
      }
      event "642 nm power (mW)": Value Change {
        n174 = event-data() -> ()  [unwired: 1 in, 6 out]
        n175 = Index Array(array=w267, index=3) -> (element=w266:T6)
        n176 = call "setLaserPower.vi"("laser power (mW)"="642 nm power (mW)", "laser"=w266) -> ()  [unwired: 1 out]
      }
      event "FW pos": Value Change {
        n177 = event-data() -> ()  [unwired: 1 in, 6 out]
        n178 = Unbundle By Name(w271) -> ("init?"=w270:i16, "FW Handle"=w269:u32)
        n179 = case shown="1" w270 {
          tunnel: w269 -> [_ w276]
          tunnel: [FALSE w273] -> _
          frame 0, Default {
          }
          frame 1 {
            n180 = local read "FW pos"() -> (w275:u16)
            n181 = To Unsigned Byte Integer(number=w275) -> (unsigned 8bit integer=w274:u8)
            n182 = call "changeFWpos.vi"("FW pos"=w274, "FWhandle"=w276) -> ("fwPosChanged"=w273:bool)
          }
        }
      }
      event "prev": Value Change {
        n183 = event-data() -> ()  [unwired: 1 in, 6 out]
        n184 = Unbundle By Name(w277) -> ("init?"=w279:i16, "FW Handle"=w278:u32)
        n185 = case shown="0, Default" w279 {
          tunnel: w278 -> [_ w281]
          frame 0, Default {
          }
          frame 1 {
            n186 = local read "FW pos"() -> (w282:u16)
            n187 = case shown="2..6" w282 {
              tunnel: w282 -> [w285 _ w287]
              tunnel: [w284 u16 6 w287] -> w280
              frame 2..6 {
                n188 = Decrement(x=w285) -> (x-1=w284:u16)
              }
              frame 1 {
              }
              frame Default {
              }
            }
            n189 = local write "FW pos"(w280) -> ()
            n190 = To Unsigned Byte Integer(number=w280) -> (unsigned 8bit integer=w283:u8)
            n191 = call "changeFWpos.vi"("FW pos"=w283, "FWhandle"=w281) -> ()  [unwired: 1 out]
          }
        }
      }
      event "next": Value Change {
        n192 = event-data() -> ()  [unwired: 1 in, 6 out]
        n193 = Unbundle By Name(w288) -> ("init?"=w290:i16, "FW Handle"=w289:u32)
        n194 = case shown="1" w290 {
          tunnel: w289 -> [_ w292]
          frame 0, Default {
          }
          frame 1 {
            n195 = local read "FW pos"() -> (w293:u16)
            n196 = case shown="1..5" w293 {
              tunnel: w293 -> [w296 _ w298]
              tunnel: [w295 u16 1 w298] -> w291
              frame 1..5 {
                n197 = Increment(x=w296) -> (x+1=w295:u16)
              }
              frame 6 {
              }
              frame Default {
              }
            }
            n198 = local write "FW pos"(w291) -> ()
            n199 = To Unsigned Byte Integer(number=w291) -> (unsigned 8bit integer=w294:u8)
            n200 = call "changeFWpos.vi"("FW pos"=w294, "FWhandle"=w292) -> ()  [unwired: 1 out]
          }
        }
      }
      event "sCMOS": Value Change {
        n201 = event-data() -> ()  [unwired: 1 in, 6 out]
        n202 = call "init_sCMOS.vi"("sCMOS_1"=TRUE) -> ("Binning"=w301:dbl, "Exposure"=w300:dbl, "sCMOS init"=w303:cluster{"init":i16, "sCMOS handle":u32})
        n203 = local write "Exposure time (s)"(w300) -> ()
        n204 = local write "sCMOS"(w303) -> ()
        n205 = To Unsigned Word Integer(number=w301) -> (unsigned 16bit integer=w302:u16)
        n206 = local write "pixel binning"(w302) -> ()
      }
      event "live stream": Value Change {
        n207 = event-data() -> ()  [unwired: 1 in, 6 out]
        n208 = local read "sCMOS"() -> (w305:cluster{"init":i16, "sCMOS handle":u32})
        n209 = Unbundle By Name(w305) -> ("init"=w304:i16)
        n210 = case shown="0, Default" w304 {
          tunnel: w308 -> [w309 w312]
          tunnel: [w309 w311] -> w307
          tunnel: w306 -> [_ w310]
          frame 0, Default {
          }
          frame 1 {
            n211 = Enqueue Element(queue=w310, element="cam1_live", error in (no error)=w312) -> (error out=w311:errorcluster)  [unwired: 1 in, 2 out]
          }
        }
      }
      event "Set exp. time": Value Change {
        n212 = event-data() -> ()  [unwired: 1 in, 6 out]
        n213 = local read "Exposure time (s)"() -> (w315:dbl)
        n214 = local read "sCMOS"() -> (w314:cluster{"init":i16, "sCMOS handle":u32})
        n215 = call "setExposureTime.vi"("sCMOS cluster"=w314, "Exposure time (s)"=w315) -> ()
      }
      event "Snap img": Value Change {
        n216 = event-data() -> ()  [unwired: 1 in, 6 out]
        n217 = local read "sCMOS"() -> (w316:cluster{"init":i16, "sCMOS handle":u32})
        n218 = call "snapImgFULL.vi"("Index"="Index", "filename"="filename", "Base path"="Base path", "sCMOS cluster"=w316) -> ("Full file"=→"Appended path":path)
        n219 = Increment(x="Index") -> (x+1=w318:i32)
        n220 = local write "Index"(w318) -> ()
      }
      event "pixel binning": Value Change {
        n221 = event-data() -> ()  [unwired: 1 in, 6 out]
        n222 = local read "sCMOS"() -> (w322:cluster{"init":i16, "sCMOS handle":u32})
        n223 = call "binPixels.vi"("pixel binning"="pixel binning", "sCMOS cluster"=w322) -> ()
        n224 = To Double Precision Float(number="No. pix") -> (double precision float=w329:dbl)
        n225 = To Double Precision Float(number="pixel binning") -> (double precision float=w327:dbl)
        n226 = Multiply(x=w327, y="scmos pixel size (um)") -> (x*y=w325:dbl)
        n227 = Divide(x=w329, y=w327) -> (x/y=w332:dbl)
        n228 = local read "Mag"() -> (w324:dbl)
        n229 = To Unsigned Word Integer(number=w332) -> (unsigned 16bit integer=→"No. of pix":u16)
        n230 = Divide(x=w325, y=w324) -> (x/y=→"Img. pixel size":dbl)
      }
      event "set init xy pos": Value Change {
        n231 = event-data() -> ()  [unwired: 1 in, 6 out]
        n232 = local read "y (mm)"() -> (w341:dbl)
        "y1" <- w341
        n233 = local read "x (mm)"() -> (w333:dbl)
        "x1" <- w333
        n234 = local read "Lat y inc (mm)"() -> (w342:dbl)
        n235 = local read "Lat x inc (mm)"() -> (w335:dbl)
        n236 = local read "y2"() -> (w340:dbl)
        n237 = local read "x2"() -> (w334:dbl)
        n238 = call "incNoStepsAcq.vi"("finPos"=w334, "initPos"=w333, "inp inc (mm)"=w335) -> ("no steps"=w336:i32, "out inc (mm)"=w339:dbl)
        n239 = call "incNoStepsAcq.vi"("finPos"=w340, "initPos"=w341, "inp inc (mm)"=w342) -> ("no steps"=w337:i32, "out inc (mm)"=w338:dbl)
        n240 = local write "Lat y inc (mm)"(w338) -> ()
        n241 = local write "no y steps"(w337) -> ()
        n242 = local write "Lat x inc (mm)"(w339) -> ()
        n243 = local write "no x steps"(w336) -> ()
      }
      event "set fin xy pos": Value Change {
        n244 = event-data() -> ()  [unwired: 1 in, 6 out]
        n245 = local read "Lat y inc (mm)"() -> (w349:dbl)
        n246 = local read "Lat x inc (mm)"() -> (w352:dbl)
        n247 = local read "x (mm)"() -> (w350:dbl)
        "x2" <- w350
        n248 = local read "y (mm)"() -> (w347:dbl)
        "y2" <- w347
        n249 = local read "y1"() -> (w348:dbl)
        n250 = local read "x1"() -> (w351:dbl)
        n251 = call "incNoStepsAcq.vi"("finPos"=w350, "initPos"=w351, "inp inc (mm)"=w352) -> ("no steps"=w345:i32, "out inc (mm)"=w346:dbl)
        n252 = call "incNoStepsAcq.vi"("finPos"=w347, "initPos"=w348, "inp inc (mm)"=w349) -> ("no steps"=w343:i32, "out inc (mm)"=w344:dbl)
        n253 = local write "Lat x inc (mm)"(w346) -> ()
        n254 = local write "no x steps"(w345) -> ()
        n255 = local write "Lat y inc (mm)"(w344) -> ()
        n256 = local write "no y steps"(w343) -> ()
      }
      event "mov init xy": Value Change {
        n257 = event-data() -> ()  [unwired: 1 in, 6 out]
        n258 = local read "x1"() -> (w353:dbl)
        n259 = local read "y1"() -> (w354:dbl)
        n260 = call "movXY.vi"("y pos (mm)"=w354, "x pos (mm)"=w353, "xy cluster"=w355) -> ()
      }
      event "mov fin xy": Value Change {
        n261 = event-data() -> ()  [unwired: 1 in, 6 out]
        n262 = local read "x2"() -> (w357:dbl)
        n263 = local read "y2"() -> (w358:dbl)
        n264 = call "movXY.vi"("y pos (mm)"=w358, "x pos (mm)"=w357, "xy cluster"=w356) -> ()
      }
      event "set init z": Value Change {
        n265 = event-data() -> ()  [unwired: 1 in, 6 out]
        n266 = local read "z (mm)"() -> (w361:dbl)
        "z1" <- w361
        n267 = local read "z inc (mm)"() -> (w363:dbl)
        n268 = local read "z2"() -> (w362:dbl)
        n269 = call "incNoStepsAcq.vi"("finPos"=w362, "initPos"=w361, "inp inc (mm)"=w363) -> ("no steps"=w360:i32, "out inc (mm)"=w359:dbl)
        n270 = local write "z inc (mm)"(w359) -> ()
        n271 = local write "no z imgs (acq)"(w360) -> ()
        n272 = local write "no z steps"(w360) -> ()
        n273 = call "mmToUm.vi"("distance (mm)"=w359) -> ("distance (um)"=w365:dbl)
        n274 = Absolute Value(x=w365) -> (abs(x)=w364:dbl)
        n275 = local write "z inc (um)"(w364) -> ()
      }
      event "set fin z": Value Change {
        n276 = event-data() -> ()  [unwired: 1 in, 6 out]
        n277 = local read "z inc (mm)"() -> (w370:dbl)
        n278 = local read "z (mm)"() -> (w368:dbl)
        "z2" <- w368
        n279 = local read "z1"() -> (w369:dbl)
        n280 = call "incNoStepsAcq.vi"("finPos"=w368, "initPos"=w369, "inp inc (mm)"=w370) -> ("no steps"=w367:i32, "out inc (mm)"=w366:dbl)
        n281 = local write "z inc (mm)"(w366) -> ()
        n282 = local write "no z imgs (acq)"(w367) -> ()
        n283 = local write "no z steps"(w367) -> ()
        n284 = call "mmToUm.vi"("distance (mm)"=w366) -> ("distance (um)"=w372:dbl)
        n285 = Absolute Value(x=w372) -> (abs(x)=w371:dbl)
        n286 = local write "z inc (um)"(w371) -> ()
      }
      event "mov init z": Value Change {
        n287 = event-data() -> ()  [unwired: 1 in, 6 out]
        n288 = Unbundle By Name(w376) -> ("System no."=w375:i32, "zIdx"=w374:i32)
        n289 = local read "z1"() -> (w373:dbl)
        n290 = call "moveStageABS.vi"("absolute pos (mm)"=w373, "axisIdx"=w374, "System no."=w375) -> ()  [unwired: 1 out]
      }
      event "mov fin z": Value Change {
        n291 = event-data() -> ()  [unwired: 1 in, 6 out]
        n292 = Unbundle By Name(w380) -> ("System no."=w379:i32, "zIdx"=w378:i32)
        n293 = local read "z2"() -> (w377:dbl)
        n294 = call "moveStageABS.vi"("absolute pos (mm)"=w377, "axisIdx"=w378, "System no."=w379) -> ()  [unwired: 1 out]
      }
      event "Read acq vals": Value Change {
        n295 = event-data() -> ()  [unwired: 1 in, 6 out]
      }
      event "Save acq vals": Value Change {
        n296 = event-data() -> ()  [unwired: 1 in, 6 out]
      }
      event "z inc (um)": Value Change {
        n297 = event-data() -> ()  [unwired: 1 in, 6 out]
        n298 = call "umTomm.vi"("distance (um)"="z inc (um)") -> ("distance (mm)"=w385:dbl)
        n299 = local read "z1"() -> (w384:dbl)
        n300 = local read "z2"() -> (w383:dbl)
        n301 = call "incNoStepsAcq.vi"("finPos"=w383, "initPos"=w384, "inp inc (mm)"=w385) -> ("no steps"=w381:i32, "out inc (mm)"=w382:dbl)
        n302 = local write "z inc (mm)"(w382) -> ()
        n303 = local write "no z steps"(w381) -> ()
        n304 = local write "no z imgs (acq)"(w381) -> ()
      }
      event "no z steps": Value Change {
        n305 = event-data() -> ()  [unwired: 1 in, 6 out]
        n306 = local read "z2"() -> (w390:dbl)
        n307 = local read "z1"() -> (w391:dbl)
        n308 = local write "no z imgs (acq)"("no z steps") -> ()
        n309 = call "calcInc.vi"("no. steps"="no z steps", "init pos (mm)"=w391, "fin pos (mm)"=w390) -> ("inc (mm)"=w388:dbl)
        n310 = local write "z inc (mm)"(w388) -> ()
        n311 = call "mmToUm.vi"("distance (mm)"=w388) -> ("distance (um)"=w392:dbl)
        n312 = Absolute Value(x=w392) -> (abs(x)=w389:dbl)
        n313 = local write "z inc (um)"(w389) -> ()
      }
      event "% FOV overlap": Value Change {
        n314 = event-data() -> ()  [unwired: 1 in, 6 out]
        n315 = local read "FOV (mm)"() -> (w402:dbl)
        n316 = call "calcLatInc.vi"("FOV (mm)"=w402, "% FOV overlap"="% FOV overlap") -> ("Lateral increment (mm)"=w396:dbl)
        n317 = local read "x1"() -> (w397:dbl)
        n318 = local read "x2"() -> (w395:dbl)
        n319 = local read "y1"() -> (w401:dbl)
        n320 = local read "y2"() -> (w400:dbl)
        n321 = call "incNoStepsAcq.vi"("finPos"=w395, "initPos"=w397, "inp inc (mm)"=w396) -> ("no steps"=→"no x steps":i32, "out inc (mm)"=→"Lat x inc (mm)":dbl)
        n322 = call "incNoStepsAcq.vi"("finPos"=w400, "initPos"=w401, "inp inc (mm)"=w396) -> ("no steps"=→"no y steps":i32, "out inc (mm)"=→"Lat y inc (mm)":dbl)
      }
      event "setupAcq": Value Change {
        n323 = event-data() -> ()  [unwired: 1 in, 6 out]
        n324 = local read "Acquiring?"() -> (w431:bool)
        n325 = local read "Base path"() -> (w413:path)
        n326 = local read "488 filter"() -> (w429:u8)
        n327 = local read "561 filter"() -> (w428:u8)
        n328 = local read "642 filter"() -> (w427:u8)
        n329 = local read "405 filter"() -> (w430:u8)
        n330 = Concatenate Strings("*" ("string"), "dcimg" ("string")) -> (w412:string)
        n331 = case shown="True" w431 {
          frame False {
          }
          frame True {
            "stop live view" <- TRUE ("stop live view")
          }
        }
        n332 = List Folder(path=w413, pattern=w412) -> (filenames=w409:string[])  [unwired: 2 in, 3 out]
        n333 = Array Size(array=w409) -> (size(s)=w406:i32)
        n334 = call "acqComponentsInit_v3.vi"("XY stage"=w416, "Z stage"=w417, "Filter wheel init"=w418, "LSFM_3 lasers"=w414, "405 nm (aq)"="405", "405 filter"=w430, "488 nm (aq)"="488", "488 filter"=w429, "561 nm (aq)"="561", "561 filter"=w428, "642 nm (aq)"="642", "642 filter"=w427) -> ("corrCompsInit?"=w407:i16, "noColours"=w415:i32, "FWpos"=→"acqFW":u8[], "acqLaserCOM"=→"acqLaserCOM":refnum<visa-resource-name>[], "acqLaserOff"=→"acqLaserOff":string[], "acqLaserOn"=→"acqLaserOn":string[])  [unwired: 2 in]
        "no colours" <- w415
        n335 = Equal To 0?(x=w406) -> (x = 0?=w405:bool)
        n336 = Boolean To (0,1)(Boolean=w405) -> (0, 1=w404:i16)
        n337 = case shown="0, Default" w404 {
          frame 0, Default {
            n338 = call "errorMessage.vi"("messageText"="There are already images in the specifed file.\nChange the specified file or delete these images.") -> ()  [unwired: 3 out]
          }
          frame 1 {
          }
        }
        n339 = And(x=w404, y=w407) -> (x .and. y?=w408:i16)
        n340 = case shown="1" w408 {
          tunnel: w415 -> [_ _]
          frame 0, Default {
            n341 = call "errorMessage.vi"("messageText"="One or more of the required components has not been intialized correctly.") -> ()  [unwired: 3 out]
          }
          frame 1 {
            n342 = local read "acquisitionMode"() -> (w434:enum32{"stop/start  ", "cont."})
            n343 = local read "% FOV overlap"() -> (w448:i32)
            n344 = local read "z inc (mm)"() -> (w435:dbl)
            n345 = local read "FOV (mm)"() -> (w447:dbl)
            n346 = property on="testAcq" class="Bool"("DisabledEnum"=T5."Enabled" ("Disabled")) -> ()  [unwired: 2 in, 2 out]
            n347 = property on="beginAcq" class="Bool"("DisabledEnum"=T5."Enabled" ("Disabled")) -> ()  [unwired: 2 in, 2 out]
            n348 = property on="stopAcq" class="Bool"("DisabledEnum"=T5."Enabled" ("Disabled")) -> ()  [unwired: 2 in, 2 out]
            n349 = call "calcLatInc.vi"("FOV (mm)"=w447, "% FOV overlap"=w448) -> ("Lateral increment (mm)"=w443:dbl)
            n350 = local read "z1"() -> (w437:dbl)
            n351 = local read "z2"() -> (w436:dbl)
            n352 = local read "x1"() -> (w444:dbl)
            n353 = local read "x2"() -> (w442:dbl)
            n354 = local read "y1"() -> (w446:dbl)
            n355 = local read "y2"() -> (w445:dbl)
            n356 = case shown="\"cont.\"" w434 {
              tunnel: w437 -> [_ w460]
              tunnel: w435 -> [_ w459]
              tunnel: w436 -> [_ w456]
              frame "stop/start  ", Default {
              }
              frame "cont." {
                n357 = local read "opticalSectionThickness (um)"() -> (w462:dbl)
                n358 = local read "Exposure time (s)"() -> (w458:dbl)
                n359 = Multiply(x=w462, y=0.001) -> (x*y=w457:dbl)
                n360 = call "calcContZStackParams.vi"("zPosInit (mm)"=w460, "zPosFin (mm)"=w456, "zIncrement (mm)"=w459, "Exposure time (s)"=w458, "opticalSectionThickness(mm)"=w457) -> ("new zPosInit (mm)"=w455:dbl, "new zPosFin (mm)"=w454:dbl, "fine axial vel (mm/s)"=w453:dbl, "acqDelay (ms)"=w452:u32)  [unwired: 7 in]
                n361 = local write "z1"(w455) -> ()
                n362 = local write "z2"(w454) -> ()
                n363 = local write "fine axial vel (mm/s)"(w453) -> ()
                n364 = local write "acqDelay (ms)"(w452) -> ()
              }
            }
            n365 = call "incNoStepsAcq.vi"("finPos"=w442, "initPos"=w444, "inp inc (mm)"=w443) -> ("no steps"=w439:i32, "out inc (mm)"=w441:dbl)
            n366 = call "incNoStepsAcq.vi"("finPos"=w445, "initPos"=w446, "inp inc (mm)"=w443) -> ("no steps"=w438:i32, "out inc (mm)"=w440:dbl)
            n367 = local write "Lat x inc (mm)"(w441) -> ()
            n368 = local write "no x steps"(w439) -> ()
            n369 = local write "Lat y inc (mm)"(w440) -> ()
            n370 = local write "no y steps"(w438) -> ()
          }
        }
      }
      event "dcimgToStack": Value Change {
        n371 = event-data() -> ()  [unwired: 1 in, 6 out]
        n372 = flat-sequence {
          tunnel: [TRUE ("Generating tiff stacks")] -> w465
          tunnel: [w470] -> w466
          tunnel: w465 -> [w469]
          tunnel: [FALSE ("Generating tiff stacks")] -> w464
          tunnel: w466 -> [_]
          tunnel: w464 -> [w473]
          frame #0 {
          }
          frame #1 {
            n373 = local write "Generating tiff stacks"(w469) -> ()
            n374 = local read "Base path"() -> (w471:path)
            n375 = call "convertDCIMGsInFileToTifStack.vi"("fileExtension"="dcimg", "path"=w471) -> ("stackConvComplete"=w470:bool)
          }
          frame #2 {
            n376 = local write "Generating tiff stacks"(w473) -> ()
          }
        }
      }
    }
    n377 = Unbundle By Name(w126) -> ("status"=w125:bool)
    n378 = Or(x=w125, y=w128) -> (x .or. y?=w127:bool)
  }
  n379 = while {
    tunnel: w21 -> [w479]
    tunnel: w22 -> [w475]
    tunnel: w20 -> [w474]
    stop <- w476 stop-if-true
    # "consumer: acquisition and live camera"
    n380 = Dequeue Element(queue=w479) -> (element=w477:string, error out=w478:errorcluster)  [unwired: 2 in, 2 out]
    n381 = case shown="No Error" w478 {
      tunnel: w477 -> [w484 _]
      tunnel: [w483 TRUE] -> w476
      tunnel: w475 -> [w482 _]
      tunnel: w474 -> [w481 _]
      frame No Error {
        n382 = case shown="\"beginAcq\"" w484 {
          tunnel: [_ _ TRUE _] -> w483
          tunnel: w482 -> [w512 _ _ w881]
          tunnel: w481 -> [w511 _ _ w880]
          tunnel: 100 ("timeout in ms (-1)") -> [w510 _ _ _]
          frame "beginAcq" {
            n383 = flat-sequence {
              tunnel: w510 -> [w556]
              tunnel: w511 -> [w557]
              tunnel: w512 -> [w558]
              tunnel: [w558] -> w509
              tunnel: [w557] -> w508
              tunnel: [w556] -> w507
              tunnel: [w524] -> w506
              tunnel: [w525] -> w505
              tunnel: [w554] -> w504
              tunnel: [w553] -> w503
              tunnel: [w551] -> w502
              tunnel: [w516] -> w501
              tunnel: [w522] -> w500
              tunnel: [w549] -> w499
              tunnel: [w521] -> w498
              tunnel: [w533] -> w497
              tunnel: [w532] -> w496
              tunnel: [w531] -> w495
              tunnel: [w530] -> w494
              tunnel: [w529] -> w493
              tunnel: [w528] -> w492
              tunnel: [w527] -> w491
              tunnel: [w526] -> w490
              tunnel: [TRUE ("Acquisition in progress")] -> w487
              tunnel: [w514] -> w485
              tunnel: w509 -> [w606]
              tunnel: w508 -> [w605]
              tunnel: w507 -> [w604]
              tunnel: w506 -> [w579]
              tunnel: w505 -> [w578]
              tunnel: w504 -> [w603]
              tunnel: w503 -> [w598]
              tunnel: w502 -> [w596]
              tunnel: w501 -> [w595]
              tunnel: w500 -> [w594]
              tunnel: w499 -> [w593]
              tunnel: w498 -> [w591]
              tunnel: w497 -> [w590]
              tunnel: w496 -> [w589]
              tunnel: w495 -> [w588]
              tunnel: w494 -> [w587]
              tunnel: w493 -> [w583]
              tunnel: w492 -> [w582]
              tunnel: w491 -> [w581]
              tunnel: w490 -> [w580]
              tunnel: [w579] -> w489
              tunnel: [w578] -> w488
              tunnel: w487 -> [w576]
              tunnel: [w575] -> w486
              tunnel: w485 -> [w574]
              tunnel: w489 -> [w863]
              tunnel: w488 -> [w864]
              tunnel: w486 -> [w866]
              frame #0 {
                n384 = local read "Acquiring?"() -> (w543:bool)
                n385 = local read "z inc (mm)"() -> (w522:dbl)
                n386 = case shown="True" w543 {
                  frame False {
                  }
                  frame True {
                    n387 = local write "stop live view"(TRUE ("stop live view")) -> ()
                  }
                }
                n388 = local read "z1"() -> (w550:dbl)
                n389 = local read "z2"() -> (w515:dbl)
                n390 = case shown="\"cont.\"" "acquisitionMode" {
                  tunnel: [w561 w566] -> w551
                  tunnel: [w562 w565] -> w516
                  tunnel: w550 -> [w562 w571]
                  tunnel: w522 -> [_ w570]
                  tunnel: w515 -> [w560 w568]
                  tunnel: [w560 w564] -> w514
                  frame "stop/start  ", Default {
                    n391 = local read "coarse axial vel (mm/s)"() -> (w561:dbl)
                  }
                  frame "cont." {
                    n392 = local read "opticalSectionThickness (um)"() -> (w573:dbl)
                    n393 = Multiply(x=w573, y=0.001) -> (x*y=w569:dbl)
                    n394 = call "calcContZStackParams.vi"("zPosInit (mm)"=w571, "zPosFin (mm)"=w568, "zIncrement (mm)"=w570, "Exposure time (s)"="Exposure time (s)", "opticalSectionThickness(mm)"=w569) -> ("new zPosInit (mm)"=w565:dbl, "new zPosFin (mm)"=w564:dbl, "fine axial vel (mm/s)"=w566:dbl, "acqDelay (ms)"=→"acqDelay (ms)":u32)  [unwired: 7 in]
                    "fine axial vel (mm/s)" <- w566
                  }
                }
                n395 = local read "% FOV overlap"() -> (w544:i32)
                n396 = local read "FOV (mm)"() -> (w545:dbl)
                n397 = local read "initLasers"() -> (w513:T1)
                n398 = local read "642 filter"() -> (w534:u8)
                n399 = local read "488 filter"() -> (w536:u8)
                n400 = local read "561 filter"() -> (w535:u8)
                n401 = local read "405 filter"() -> (w537:u8)
                n402 = local read "642"() -> (w540:bool)
                n403 = local read "561"() -> (w539:bool)
                n404 = local read "488"() -> (w538:bool)
                n405 = local read "405"() -> (w541:bool)
                n406 = call "calcLatInc.vi"("FOV (mm)"=w545, "% FOV overlap"=w544) -> ("Lateral increment (mm)"=w547:dbl)
                n407 = local read "x1"() -> (w529:dbl)
                n408 = local read "y1"() -> (w528:dbl)
                n409 = local read "x2"() -> (w548:dbl)
                n410 = local read "y2"() -> (w546:dbl)
                n411 = call "acqInitLasersFW.vi"("LSFM_3 lasers"=w513, "405 nm (aq)"=w541, "405 filter"=w537, "488 nm (aq)"=w538, "488 filter"=w536, "561 nm (aq)"=w539, "561 filter"=w535, "642 nm (aq)"=w540, "642 filter"=w534) -> ("FWpos"=w521:u8[], "acqLaserCOM"=w533:refnum<visa-resource-name>[], "acqLaserOn"=w532:string[], "acqLaserOff"=w531:string[])  [unwired: 7 in]
                n412 = call "incNoStepsAcq.vi"("finPos"=w514, "initPos"=w516, "inp inc (mm)"=w522) -> ("no steps"=w518:i32, "out inc (mm)"=w542:dbl)
                n413 = local read "Base path"() -> (w555:path)
                n414 = call "incNoStepsAcq.vi"("finPos"=w548, "initPos"=w529, "inp inc (mm)"=w547) -> ("no steps"=w520:i32, "out inc (mm)"=w527:dbl)
                n415 = call "incNoStepsAcq.vi"("finPos"=w546, "initPos"=w528, "inp inc (mm)"=w547) -> ("no steps"=w519:i32, "out inc (mm)"=w526:dbl)
                n416 = local write "z inc (mm)"(w542) -> ()
                n417 = Array Size(array=w521) -> (size(s)=w517:i32)
                n418 = local read "Filter wheel"() -> (w549:cluster{"FW Handle":u32, "init?":i16})
                n419 = local read "XY stage"() -> (w530:T3)
                n420 = local read "sCMOS"() -> (w553:cluster{"init":i16, "sCMOS handle":u32})
                n421 = local read "Z stage"() -> (w554:T2)
                n422 = call "createFilenameArray_slim.vi"("no x steps"=w520, "no y steps"=w519, "no z steps"=w518, "No colours"=w517, "Base path"=w555) -> ("stackFnameArray"=w525:path[][][], "frameFilenameArray"=w524:path[][][][])
              }
              frame #1 {
                n423 = Unbundle By Name(w598) -> ("sCMOS handle"=w597:u32)
                n424 = Unbundle By Name(w593) -> ("FW Handle"=w592:u32)
                n425 = Unbundle By Name(w603) -> ("System no."=w602:i32, "zIdx"=w601:i32)
                n426 = Unbundle By Name(w587) -> ("System no."=w586:i32, "xIdx"=w585:i32, "yIdx"=w584:i32)
                n427 = local read "coarse axial vel (mm/s)"() -> (w600:dbl)
                n428 = local read "acquisitionMode"() -> (w577:enum32{"stop/start  ", "cont."})
                n429 = local read "acqDelay (ms)"() -> (w599:u32)
                n430 = for {
                  tunnel: w606 -> [w659]
                  tunnel: w604 -> [w657]
                  shift-right: [w653] -> _
                  shift-left: w605 -> [w658]
                  tunnel: w594 -> [w649]
                  tunnel: w597 -> [w647]
                  tunnel: w579 -> [w645] mode=indexing
                  tunnel: w602 -> [w642]
                  tunnel: w601 -> [w641]
                  tunnel: w595 -> [w643]
                  tunnel: w596 -> [w638]
                  tunnel: w600 -> [w637]
                  tunnel: w577 -> [w636]
                  tunnel: w574 -> [w635]
                  tunnel: w599 -> [w634]
                  tunnel: w592 -> [w633]
                  tunnel: w591 -> [w632] mode=indexing
                  tunnel: w590 -> [w631] mode=indexing
                  tunnel: w589 -> [w630] mode=indexing
                  tunnel: w588 -> [w627] mode=indexing
                  tunnel: w586 -> [w624]
                  tunnel: w585 -> [w623]
                  tunnel: w584 -> [w622]
                  tunnel: w583 -> [w621]
                  tunnel: w582 -> [w620]
                  tunnel: w581 -> [w615]
                  tunnel: w580 -> [w608]
                  tunnel: [FALSE ("Acquisition in progress")] -> w575
                  stop <- w654 stop-if-true
                  n431 = Wait on Notification(notifier=w659, timeout in ms (-1)=w657, error in (no error)=w658) -> (timed out?=w655:bool, error out=w653:errorcluster)  [unwired: 1 in, 2 out]
                  n432 = flat-sequence {
                    tunnel: w657 -> [w681]
                    tunnel: w658 -> [w682]
                    tunnel: w659 -> [w683]
                    tunnel: [w683] -> w652
                    tunnel: [w682] -> w651
                    tunnel: [w681] -> w650
                    tunnel: w649 -> [w680]
                    tunnel: [w680] -> w648
                    tunnel: w647 -> [w679]
                    tunnel: [w679] -> w646
                    tunnel: w645 -> [w678]
                    tunnel: [w678] -> w644
                    tunnel: w643 -> [w674]
                    tunnel: w642 -> [w677]
                    tunnel: w641 -> [w676]
                    tunnel: [w675] -> w640
                    tunnel: [w674] -> w639
                    tunnel: w633 -> [w673]
                    tunnel: w632 -> [w672]
                    tunnel: w631 -> [w670]
                    tunnel: w630 -> [w671]
                    tunnel: [w670] -> w628
                    tunnel: w627 -> [w669]
                    tunnel: [w669] -> w625
                    tunnel: w624 -> [w664]
                    tunnel: w624 -> [w660]
                    tunnel: w623 -> [w663]
                    tunnel: w622 -> [w661]
                    tunnel: w621 -> [w662]
                    tunnel: w620 -> [w668]
                    tunnel: [w667] -> w619
                    tunnel: [w666] -> w618
                    tunnel: [w663] -> w617
                    tunnel: [w664] -> w616
                    tunnel: w615 -> [w665]
                    tunnel: [w665] -> w614
                    tunnel: [w664] -> w613
                    tunnel: [w663] -> w612
                    tunnel: [w662] -> w611
                    tunnel: [w661] -> w610
                    tunnel: [w660] -> w609
                    tunnel: w652 -> [w708]
                    tunnel: w651 -> [w707]
                    tunnel: w650 -> [w706]
                    tunnel: w648 -> [w705]
                    tunnel: w646 -> [w704]
                    tunnel: w644 -> [w703]
                    tunnel: w642 -> [w702]
                    tunnel: w641 -> [w701]
                    tunnel: w640 -> [_]
                    tunnel: w639 -> [w700]
                    tunnel: w638 -> [w699]
                    tunnel: w637 -> [w698]
                    tunnel: w636 -> [w697]
                    tunnel: w635 -> [w696]
                    tunnel: w634 -> [w695]
                    tunnel: [w694] -> w629
                    tunnel: w628 -> [w694]
                    tunnel: [w693] -> w626
                    tunnel: w625 -> [w693]
                    tunnel: w619 -> [_]
                    tunnel: w618 -> [_]
                    tunnel: w617 -> [w692]
                    tunnel: w616 -> [w691]
                    tunnel: w614 -> [w690]
                    tunnel: w613 -> [w689]
                    tunnel: w612 -> [w688]
                    tunnel: w611 -> [w687]
                    tunnel: w610 -> [w686]
                    tunnel: w609 -> [w685]
                    tunnel: w608 -> [w684]
                    tunnel: w629 -> [w862]
                    tunnel: w626 -> [w861]
                    frame #0 {
                      n433 = call "changeFWposAcq.vi"("FW pos"=w672, "FWhandle"=w673) -> ()
                      n434 = call "writeToSerialAcq.vi"("Cmmd"=w671, "input COM Port"=w670) -> ()
                      n435 = call "moveStageABS.vi"("absolute pos (mm)"=w674, "axisIdx"=w676, "System no."=w677) -> ("Stopped"=w675:bool)
                      n436 = call "moveStageABS.vi"("absolute pos (mm)"=w662, "axisIdx"=w663, "System no."=w664) -> ("Stopped"=w667:bool)
                      n437 = call "moveStageABS.vi"("absolute pos (mm)"=w668, "axisIdx"=w661, "System no."=w660) -> ("Stopped"=w666:bool)
                    }
                    frame #1 {
                      n438 = for {
                        tunnel: w708 -> [w737]
                        tunnel: w706 -> [w736]
                        shift-right: [w734] -> _
                        shift-left: w707 -> [w735]
                        tunnel: w705 -> [w730]
                        tunnel: w704 -> [w729]
                        tunnel: w703 -> [w728] mode=indexing
                        tunnel: w702 -> [w727]
                        tunnel: w701 -> [w726]
                        tunnel: w702 -> [w725]
                        tunnel: w701 -> [w724]
                        tunnel: w700 -> [w723]
                        tunnel: w699 -> [w722]
                        tunnel: w698 -> [w721]
                        tunnel: w697 -> [w720]
                        tunnel: w696 -> [w719]
                        tunnel: w695 -> [w718]
                        tunnel: w692 -> [w717]
                        tunnel: w691 -> [w716]
                        tunnel: w690 -> [w715]
                        tunnel: w689 -> [w714]
                        tunnel: w688 -> [w713]
                        tunnel: w687 -> [w712]
                        tunnel: w686 -> [w711]
                        tunnel: w685 -> [w710]
                        tunnel: w684 -> [w709]
                        stop <- w731 stop-if-true
                        n439 = Wait on Notification(notifier=w737, timeout in ms (-1)=w736, error in (no error)=w735) -> (timed out?=w733:bool, error out=w734:errorcluster)  [unwired: 1 in, 2 out]
                        n440 = flat-sequence {
                          tunnel: w737 -> [w756]
                          tunnel: w736 -> [w755]
                          tunnel: w735 -> [w754]
                          tunnel: w730 -> [w753]
                          tunnel: w729 -> [w752]
                          tunnel: w728 -> [w751]
                          tunnel: w727 -> [w750]
                          tunnel: w726 -> [w749]
                          tunnel: w725 -> [w748]
                          tunnel: w724 -> [w747]
                          tunnel: w723 -> [w746]
                          tunnel: w722 -> [w745]
                          tunnel: w721 -> [w744]
                          tunnel: w720 -> [w743]
                          tunnel: w719 -> [w742]
                          tunnel: w718 -> [w741]
                          tunnel: w717 -> [w740]
                          tunnel: w716 -> [w739]
                          tunnel: w715 -> [w738]
                          tunnel: [w860] -> _
                          tunnel: [w859] -> _
                          tunnel: w714 -> [w858]
                          tunnel: w713 -> [w857]
                          tunnel: w712 -> [w856]
                          tunnel: w711 -> [w855]
                          tunnel: w710 -> [w854]
                          tunnel: w709 -> [w853]
                          frame #0 {
                            n441 = for {
                              tunnel: w756 -> [w794]
                              shift-right: [w789] -> _
                              shift-left: w754 -> [w792]
                              tunnel: w755 -> [w793]
                              tunnel: w753 -> [w787]
                              tunnel: w752 -> [w775]
                              tunnel: w751 -> [w786] mode=indexing
                              tunnel: w750 -> [w785]
                              tunnel: w749 -> [w784]
                              tunnel: w748 -> [w783]
                              tunnel: w747 -> [w782]
                              tunnel: w746 -> [w781]
                              tunnel: w745 -> [w780]
                              tunnel: w744 -> [w779]
                              tunnel: w743 -> [w778]
                              tunnel: w742 -> [w777]
                              tunnel: w741 -> [w776]
                              tunnel: w740 -> [w774]
                              tunnel: w739 -> [w773]
                              tunnel: w738 -> [w772]
                              stop <- w788 stop-if-true
                              n442 = Wait on Notification(notifier=w794, timeout in ms (-1)=w793, error in (no error)=w792) -> (timed out?=w790:bool, error out=w789:errorcluster)  [unwired: 1 in, 2 out]
                              n443 = flat-sequence {
                                tunnel: w775 -> [w796]
                                tunnel: w776 -> [w797]
                                tunnel: w777 -> [w798]
                                tunnel: w778 -> [w799]
                                tunnel: w779 -> [w800]
                                tunnel: w780 -> [w801]
                                tunnel: w784 -> [w802]
                                tunnel: w785 -> [w803]
                                tunnel: w786 -> [w804]
                                tunnel: w787 -> [w805]
                                tunnel: w792 -> [w806]
                                tunnel: w793 -> [w807]
                                tunnel: w794 -> [w808]
                                tunnel: [w808] -> w771
                                tunnel: [w807] -> w770
                                tunnel: [w806] -> w769
                                tunnel: [w805] -> w768
                                tunnel: [w804] -> w767
                                tunnel: [w803] -> w766
                                tunnel: [w802] -> w765
                                tunnel: [w801] -> w764
                                tunnel: [w800] -> w763
                                tunnel: [w799] -> w762
                                tunnel: [w798] -> w761
                                tunnel: [w797] -> w760
                                tunnel: [w796] -> w759
                                tunnel: [w795] -> w758
                                tunnel: w771 -> [w822]
                                tunnel: w770 -> [w821]
                                tunnel: w769 -> [w820]
                                tunnel: w768 -> [w819]
                                tunnel: w767 -> [w818]
                                tunnel: w766 -> [w817]
                                tunnel: w765 -> [w816]
                                tunnel: w764 -> [w815]
                                tunnel: w763 -> [w814]
                                tunnel: w762 -> [w813]
                                tunnel: w761 -> [w812]
                                tunnel: w760 -> [w811]
                                tunnel: w759 -> [w810]
                                tunnel: w758 -> [w809]
                                tunnel: [w809] -> w757
                                tunnel: w783 -> [w852]
                                tunnel: w782 -> [w851]
                                tunnel: w781 -> [w850]
                                tunnel: [w849] -> _
                                tunnel: w774 -> [w848]
                                tunnel: w773 -> [w847]
                                tunnel: w772 -> [w846]
                                tunnel: [w845] -> _
                                tunnel: w757 -> [w843]
                                frame #0 {
                                n444 = Tick Count (ms)() -> (millisecond timer value=w795:u32)
                                }
                                frame #1 {
                                n445 = case shown="\"stop/start  \", Default" w813 {
                                tunnel: w822 -> [_ w836]
                                tunnel: w821 -> [_ w834]
                                tunnel: w820 -> [_ w835]
                                tunnel: w819 -> [_ w837]
                                tunnel: w818 -> [w831 w840]
                                tunnel: w817 -> [w826 w839]
                                tunnel: w816 -> [w825 w838]
                                tunnel: w815 -> [w823 _]
                                tunnel: w814 -> [w830 _]
                                tunnel: w812 -> [w824 _]
                                tunnel: w811 -> [w829 _]
                                tunnel: w810 -> [w827 w833]
                                tunnel: [w832 w841] -> _
                                frame "cont." {
                                n446 = call "contMotionAcq.vi"("sCMOS handle"=w827, "fine axial vel (mm/s)"=w823, "coarse axial vel (mm/s)"=w830, "System no."=w826, "zIdx"=w825, "z2"=w824, "imgFilenames"=w831, "stageAccDelay (ms)"="stageAccDelay (ms)", "acqDelay (ms)"=w829) -> ("Controller error"=w832:bool)  [unwired: 6 in]
                                }
                                frame "stop/start  ", Default {
                                n447 = call "stopStartMotionAcq.vi"("error out"=w835, "timeout"=w834, "notifier out"=w836, "frameFilenameArray"=w840, "z inc (mm)"=w837, "zIdx"=w838, "System no."=w839, "sCMOShandle"=w833) -> ("Stopped"=w841:bool)  [unwired: 2 in]
                                }
                                }
                                }
                                frame #2 {
                                n448 = call "moveStageABS.vi"("absolute pos (mm)"=w850, "axisIdx"=w851, "System no."=w852) -> ("Stopped"=w845:bool)
                                n449 = call "moveStage.vi"("inc (mm)"=w846, "axisIdx"=w848, "System no."=w847) -> ("Stopped"=w849:bool)
                                n450 = Tick Count (ms)() -> (millisecond timer value=w844:u32)
                                n451 = Subtract(x=w844, y=w843) -> (x-y=→"acquisitionTime":u32)
                                }
                              }
                              n452 = Unbundle By Name(w789) -> ("status"=w791:bool)
                              n453 = Compound Arithmetic op=OR(invert w790, w791) -> (w788:bool)
                            }
                          }
                          frame #1 {
                            n454 = call "moveStage.vi"("inc (mm)"=w853, "axisIdx"=w855, "System no."=w854) -> ("Stopped"=w860:bool)
                            n455 = call "moveStageABS.vi"("absolute pos (mm)"=w856, "axisIdx"=w857, "System no."=w858) -> ("Stopped"=w859:bool)
                          }
                        }
                        n456 = Unbundle By Name(w734) -> ("status"=w732:bool)
                        n457 = Compound Arithmetic op=OR(invert w733, w732) -> (w731:bool)
                      }
                    }
                    frame #2 {
                      n458 = call "writeToSerialAcq.vi"("Cmmd"=w861, "input COM Port"=w862) -> ()
                    }
                  }
                  n459 = Unbundle By Name(w653) -> ("status"=w656:bool)
                  n460 = Compound Arithmetic op=OR(invert w655, w656) -> (w654:bool)
                }
                "Acquisition in progress" <- w576
              }
              frame #2 {
                n461 = local write "Acquisition in progress"(w866) -> ()
                n462 = case shown="True" "convertDcimgToTifStacks" {
                  tunnel: w864 -> [_ w867]
                  tunnel: w863 -> [_ w868]
                  frame False {
                  }
                  frame True {
                    n463 = flat-sequence {
                      tunnel: [w872] -> w869
                      tunnel: w868 -> [w871]
                      tunnel: w867 -> [w870]
                      tunnel: w869 -> [w874]
                      frame #0 {
                        n464 = call "generateTiffStacks.vi"("singleImgFname"=w871, "stackFname"=w870) -> ("stackGenerationComplete"=w872:bool)
                        n465 = local write "Generating tiff stacks"(TRUE ("Generating tiff stacks")) -> ()
                      }
                      frame #1 {
                        "Generating tiff stacks" <- w874
                      }
                    }
                  }
                }
              }
            }
          }
          frame "idle", Default {
          }
          frame "mainStop" {
            # "Stutdown process here."
          }
          frame "cam1_live" {
            w886 = 1 items=["Snap", "Sequence"] ("Capture mode")
            n466 = local read "sCMOS"() -> (w889:cluster{"init":i16, "sCMOS handle":u32})
            n467 = Unbundle By Name(w889) -> ("sCMOS handle"=w885:u32)
            n468 = call <userlib>:"tm_preparecapture.vi"("Capture mode"=w886, "Handle in"=w885) -> ("error out"=w887:errorcluster, "Buffer Info"=w884:T8, "Handle out"=w888:u32)  [unwired: 6 in, 1 out]
            n469 = call <userlib>:"tm_startcapture_b.vi"("error in (no error)"=w887, "Handle in"=w888) -> ("error out"=w882:errorcluster, "Handle out"=w883:u32)  [unwired: 8 in]
            n470 = while {
              tunnel: w884 -> [w899]
              tunnel: w883 -> [w898]
              tunnel: w882 -> [w897]
              tunnel: w881 -> [w905]
              shift-right: [w903] -> _
              shift-left: w880 -> [w904]
              tunnel: [w894] -> w877
              tunnel: [w893] -> w876
              stop <- w892 stop-if-true
              n471 = call <userlib>:"tm_waitnextframe.vi"("error in (no error)"=w897, "Handle in"=w898) -> ("error out"=w900:errorcluster, "Frame Index"=w902:i32, "Handle out"=w901:u32)  [unwired: 6 in, 1 out]
              n472 = call <userlib>:"tm_getframe_a.vi"("error in (no error)"=w900, "Frame Index"=w902, "Buffer Info"=w899, "Handle in"=w901) -> ("error out"=w893:errorcluster, "Data 16"=w895:u16[][], "Handle out"=w894:u32)  [unwired: 3 in, 2 out]
              n473 = Wait on Notification(notifier=w905, timeout in ms (-1)=100, error in (no error)=w904) -> (timed out?=w907:bool, error out=w903:errorcluster)  [unwired: 1 in, 2 out]
              n474 = local read "stop live view"() -> (w890:bool)
              n475 = case shown="True" "View stream" {
                tunnel: w895 -> [_ w914]
                frame False {
                }
                frame True {
                  n476 = call "liveCameraView.vi"("Data 16"=w914) -> ("VI Refnum"=w912:refnum<vi>)
                  n477 = invoke class="VI" method="FP.Open"(reference=w912, "Activate"=FALSE ("Activate?"), "State"=T7."Standard") -> ()  [unwired: 2 in, 5 out]
                }
              }
              n478 = Unbundle By Name(w903) -> ("status"=w906:bool)
              n479 = Compound Arithmetic op=OR(invert w907, w906, "stop live stream", w890) -> (w892:bool)
              n480 = case shown="False" w892 {
                frame False {
                }
                frame True {
                  n481 = local write "Acquiring?"(FALSE ("Acquiring?")) -> ()
                }
              }
              "Acquiring?" <- TRUE ("Acquiring?")
            }
            n482 = call <userlib>:"tm_stopcapture.vi"("error in (no error)"=w876, "Handle in"=w877) -> ("error out"=w878:errorcluster, "Handle out"=w879:u32)  [unwired: 8 in]
            n483 = call <userlib>:"tm_unpreparecapture.vi"("error in (no error)"=w878, "Handle in"=w879) -> ()  [unwired: 8 in, 2 out]
          }
        }
      }
      frame Error {
        # "Return true in any case that should stop the loop."
      }
    }
  }
  n484 = Release Queue(queue=w21, error in (no error)=w25) -> (error out=w24:errorcluster)  [unwired: 1 in, 2 out]
  n485 = Release Notifier(notifier=w22, error in (no error)=w24) -> (error out=w23:errorcluster)  [unwired: 1 in, 2 out]
  n486 = call <vilib>:"General Error Handler.vi"("error in (no error)"=w23) -> ()  [unwired: 10 in, 5 out]
